vi "RTK Multiple String Capture Software.vi"() -> ()   [LabVIEW 2009]
uses:
  <vilib>/Instr/_visa.llb/VISA Configure Serial Port (Instr).vi
  <vilib>/Instr/_visa.llb/VISA Flush IO Buffer Mask.ctl
  COM Port Control.ctl
panel:
  in  "Tab Control":T1(tab)
  in  "Update setup":bool
  in  "stop":bool
  in  "Base File Path":path caption="Base File Path (Destination that all RCVR files will be saved in)"
  in  "Time between samples (seconds)":u32 max=600 step=1
  in  "Number of hours To Collect before starting new file":u16 min=1 max=24 step=1
  in  "UPDT COM 1":bool
  in  "Use RCVR 1":bool caption="Use RCVR"
  in  "Name of RCVR 1":string caption="Name of RCVR"
  in  "COM Port 1":T2 {"data bits" min=5 max=8 step=1; "flow control" items=["None", "XON/XOFF", "RTS/CTS", "XON/XOFF & RTS/CTS", "DTR/DSR", "XON/XOFF & DTR/DSR"]}
  out "Last 10 RCVR 1":string[](array[string])
  in  "Name of RCVR 2":string caption="Name of RCVR"
  in  "UPDT COM 2":bool
  out "Last 10 RCVR 2":string[](array[string])
  in  "COM Port 2":T2 {"data bits" min=5 max=8 step=1; "flow control" items=["None", "XON/XOFF", "RTS/CTS", "XON/XOFF & RTS/CTS", "DTR/DSR", "XON/XOFF & DTR/DSR"]}
  in  "Use RCVR 2":bool caption="Use RCVR"
  in  "Name of RCVR 3":string caption="Name of RCVR"
  in  "UPDT COM 3":bool
  out "Last 10 RCVR 3":string[](array[string])
  in  "COM Port 3":T2 {"data bits" min=5 max=8 step=1; "flow control" items=["None", "XON/XOFF", "RTS/CTS", "XON/XOFF & RTS/CTS", "DTR/DSR", "XON/XOFF & DTR/DSR"]}
  in  "Use RCVR 3":bool caption="Use RCVR"
  in  "Name of RCVR 4":string caption="Name of RCVR"
  in  "UPDT COM 4":bool
  out "Last 10 RCVR 4":string[](array[string])
  in  "COM Port 4":T2 {"data bits" min=5 max=8 step=1; "flow control" items=["None", "XON/XOFF", "RTS/CTS", "XON/XOFF & RTS/CTS", "DTR/DSR", "XON/XOFF & DTR/DSR"]}
  in  "Use RCVR 4":bool caption="Use RCVR"
  in  "Name of RCVR 5":string caption="Name of RCVR"
  in  "UPDT COM 5":bool
  out "Last 10 RCVR 5":string[](array[string])
  in  "COM Port 5":T2 {"data bits" min=5 max=8 step=1; "flow control" items=["None", "XON/XOFF", "RTS/CTS", "XON/XOFF & RTS/CTS", "DTR/DSR", "XON/XOFF & DTR/DSR"]}
  in  "Use RCVR 5":bool caption="Use RCVR"
  in  "Name of RCVR 6":string caption="Name of RCVR"
  in  "UPDT COM 6":bool
  out "Last 10 RCVR 6":string[](array[string])
  in  "COM Port 6":T2 {"data bits" min=5 max=8 step=1; "flow control" items=["None", "XON/XOFF", "RTS/CTS", "XON/XOFF & RTS/CTS", "DTR/DSR", "XON/XOFF & DTR/DSR"]}
  in  "Use RCVR 6":bool caption="Use RCVR"
  in  "Name of RCVR 7":string caption="Name of RCVR"
  in  "UPDT COM 7":bool
  out "Last 10 RCVR 7":string[](array[string])
  in  "COM Port 7":T2 {"data bits" min=5 max=8 step=1; "flow control" items=["None", "XON/XOFF", "RTS/CTS", "XON/XOFF & RTS/CTS", "DTR/DSR", "XON/XOFF & DTR/DSR"]}
  in  "Use RCVR 7":bool caption="Use RCVR"
  in  "Name of RCVR 8":string caption="Name of RCVR"
  in  "UPDT COM 8":bool
  out "Last 10 RCVR 8":string[](array[string])
  in  "COM Port 8":T2 {"data bits" min=5 max=8 step=1; "flow control" items=["None", "XON/XOFF", "RTS/CTS", "XON/XOFF & RTS/CTS", "DTR/DSR", "XON/XOFF & DTR/DSR"]}
  in  "Use RCVR 8":bool caption="Use RCVR"
  in  "Name of RCVR 9":string caption="Name of RCVR"
  in  "UPDT COM 9":bool
  out "Last 10 RCVR 9":string[](array[string])
  in  "COM Port 9":T2 {"data bits" min=5 max=8 step=1; "flow control" items=["None", "XON/XOFF", "RTS/CTS", "XON/XOFF & RTS/CTS", "DTR/DSR", "XON/XOFF & DTR/DSR"]}
  in  "Use RCVR 9":bool caption="Use RCVR"
  in  "Name of RCVR 10":string caption="Name of RCVR"
  in  "UPDT COM 10":bool
  out "Last 10 RCVR 10":string[](array[string])
  in  "COM Port 10":T2 {"data bits" min=5 max=8 step=1; "flow control" items=["None", "XON/XOFF", "RTS/CTS", "XON/XOFF & RTS/CTS", "DTR/DSR", "XON/XOFF & DTR/DSR"]}
  in  "Use RCVR 10":bool caption="Use RCVR"
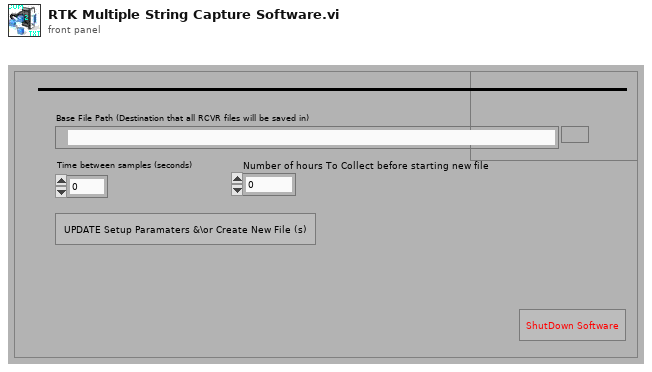
[diagram p1: front panel]
types:
  T1 = enum32{"SETUP", "RCVR 1", "RCVR 2", "RCVR 3", "RCVR 4", "RCVR 5", "RCVR 6", "RCVR 7", "RCVR 8", "RCVR 9", "RCVR 10"}
  T2 = typedef "COM Port Control.ctl" = cluster{"flow control":u16, "COM Port":refnum<visa-resource-name>, "parity":enum16{"None", "Odd", "Even", "Mark", "Space"}, "data bits":u16, "baud rate":u32}
  T3 = typedef "VISA Flush IO Buffer Mask.ctl" = u16
  T4 = enum32{"invalid app kind", "Development System", "Run Time System", "Student Edition", "Embedded LabVIEW", "Evaluation", "Custom"}
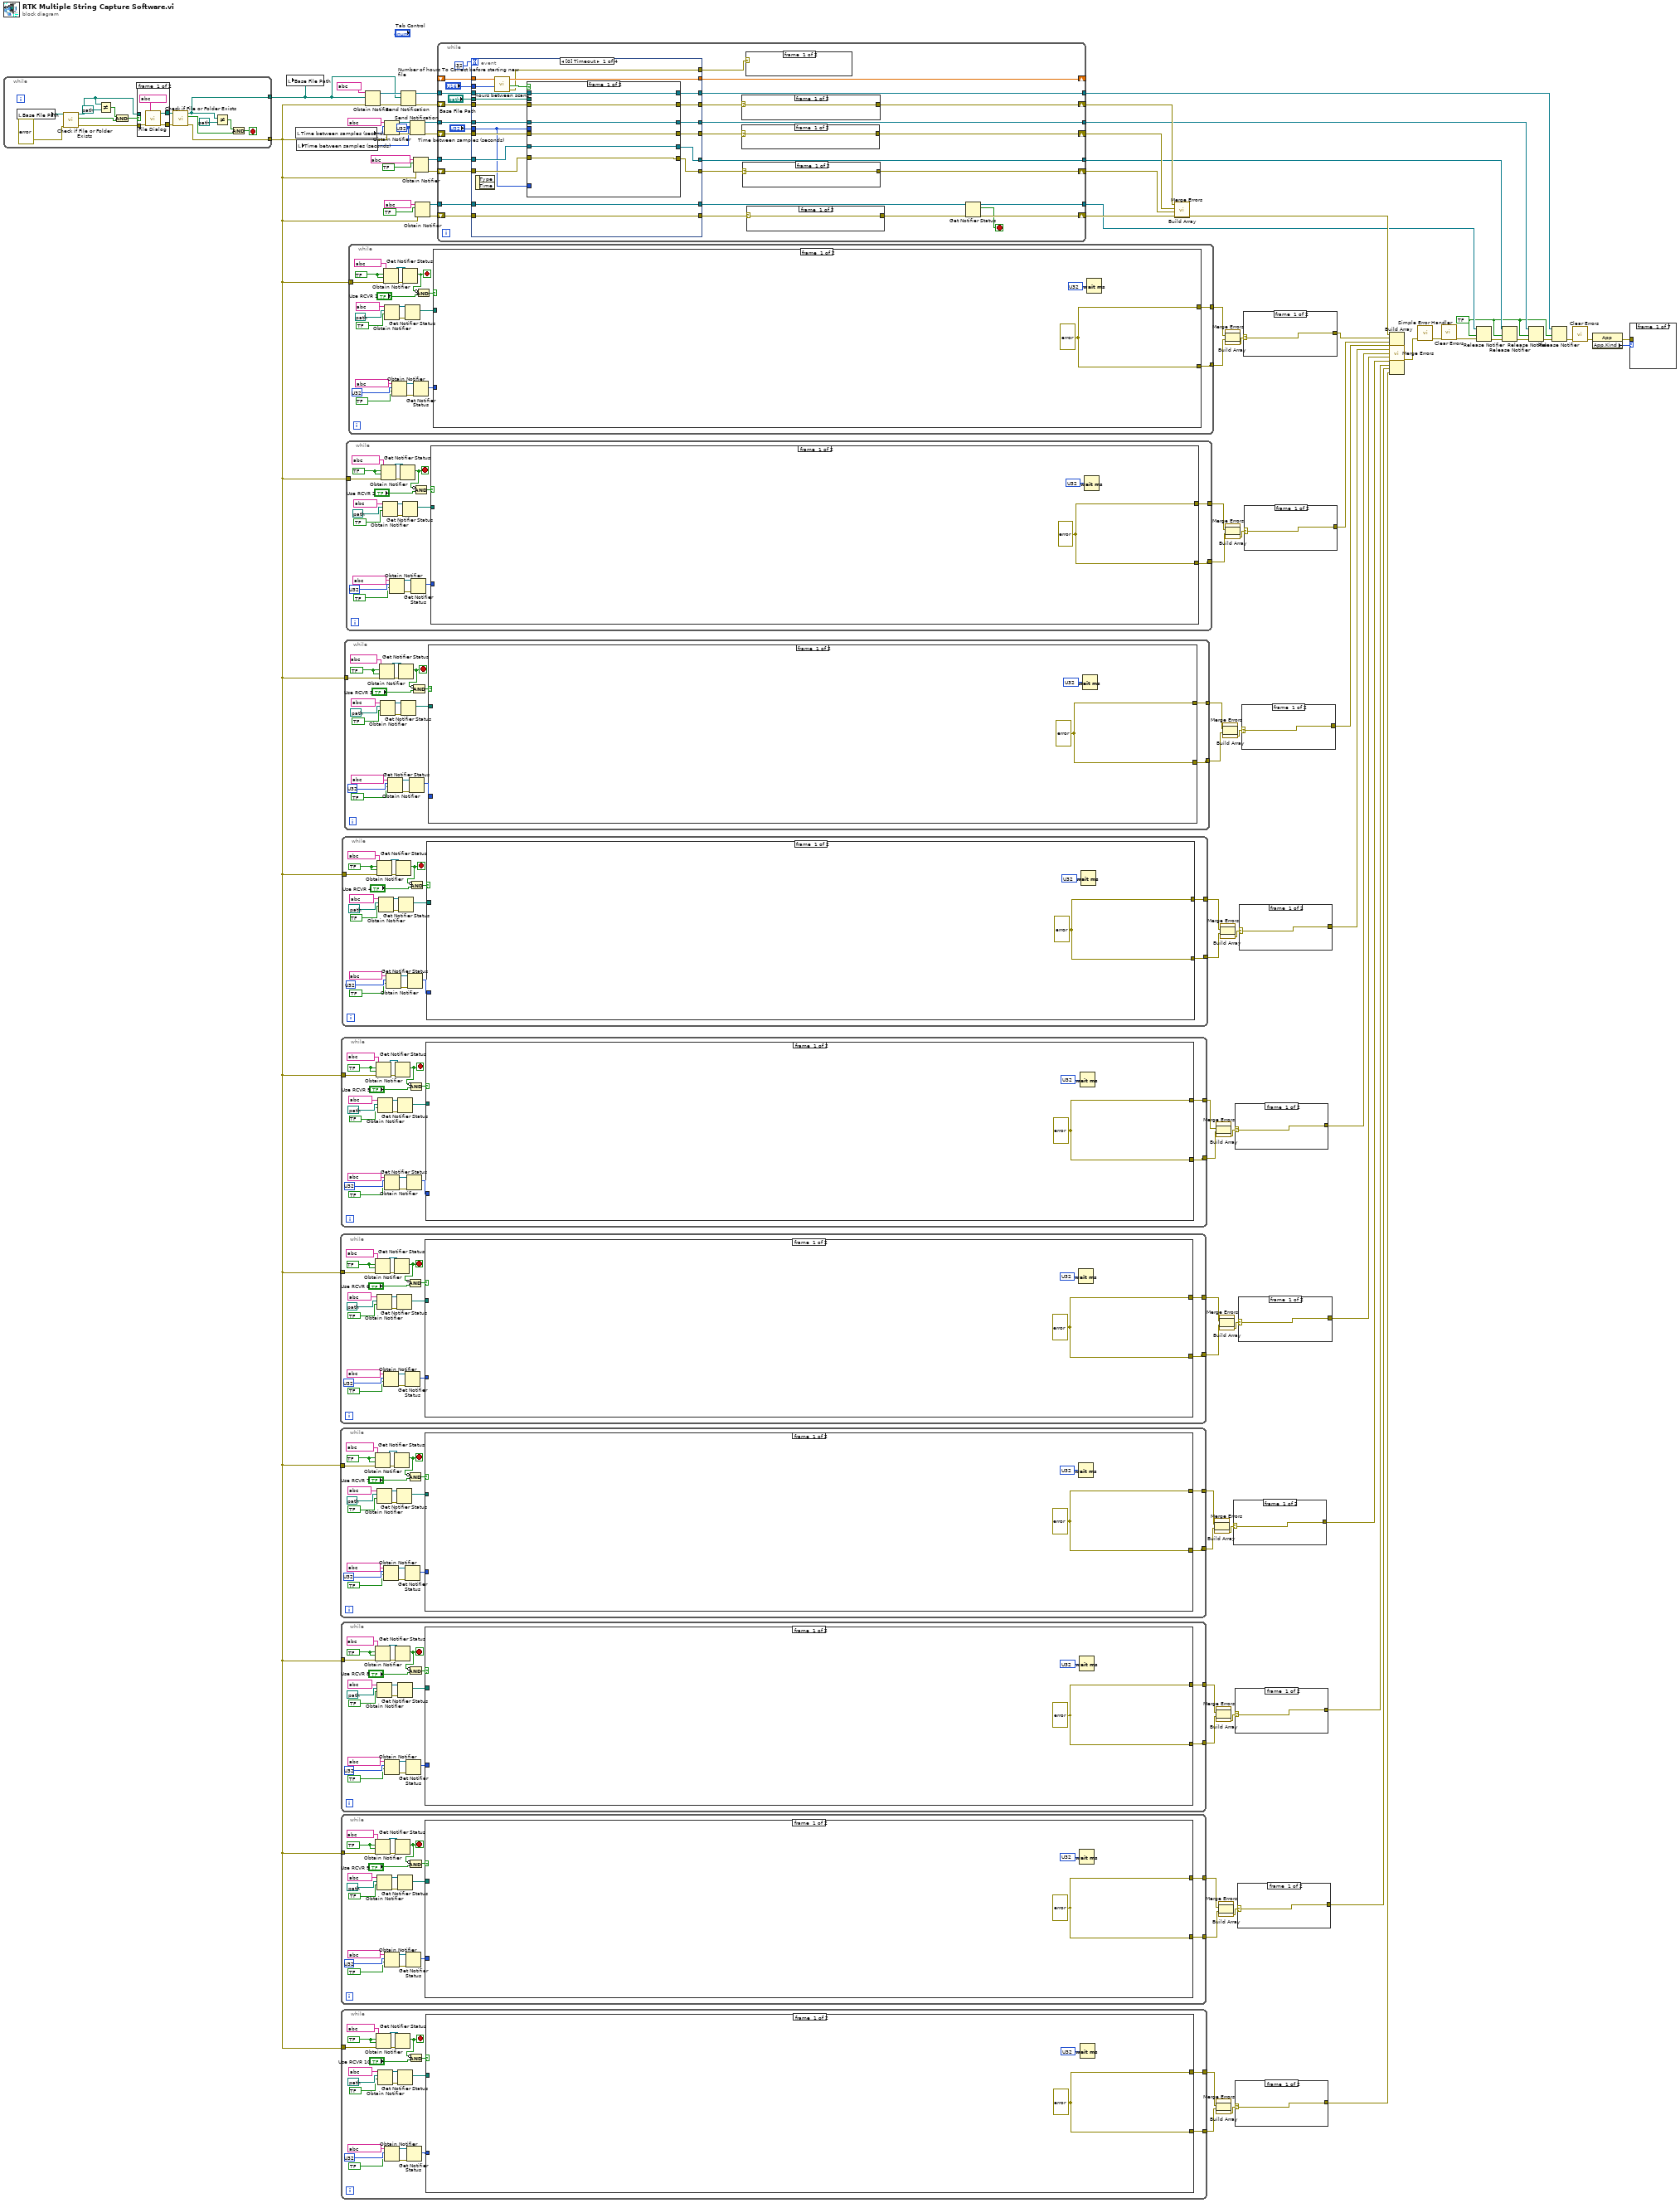
[diagram p0: block diagram]
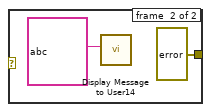
[diagram p2: hidden frame]
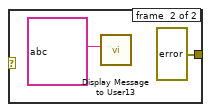
[diagram p3: hidden frame]
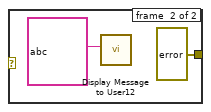
[diagram p4: hidden frame]
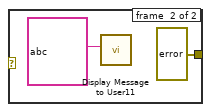
[diagram p5: hidden frame]
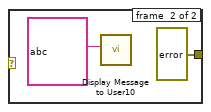
[diagram p6: hidden frame]
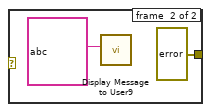
[diagram p7: hidden frame]
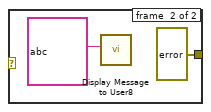
[diagram p8: hidden frame]
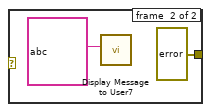
[diagram p9: hidden frame]
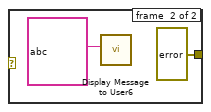
[diagram p10: hidden frame]
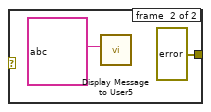
[diagram p11: hidden frame]
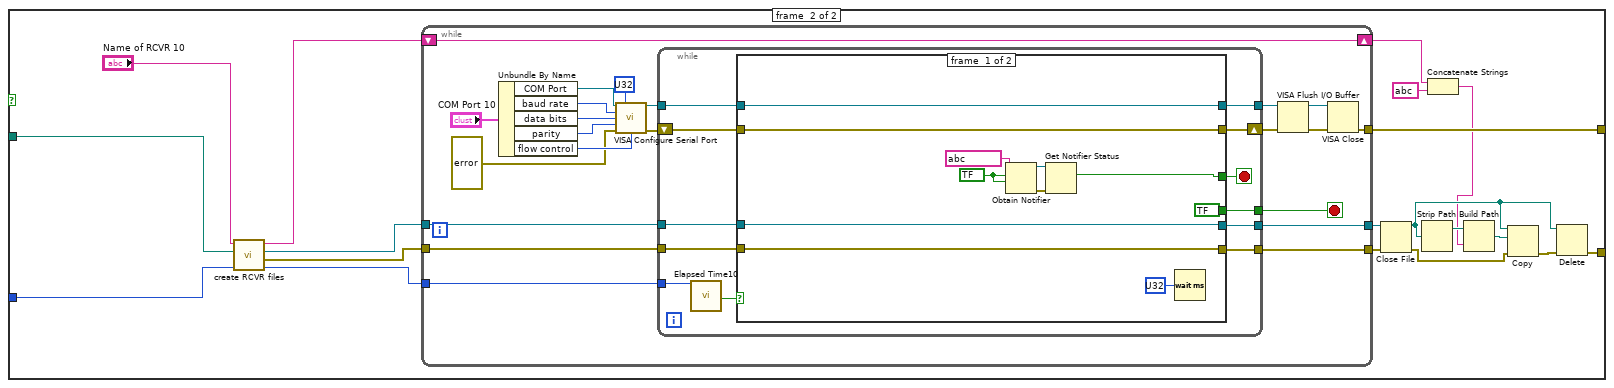
[diagram p12: hidden frame]
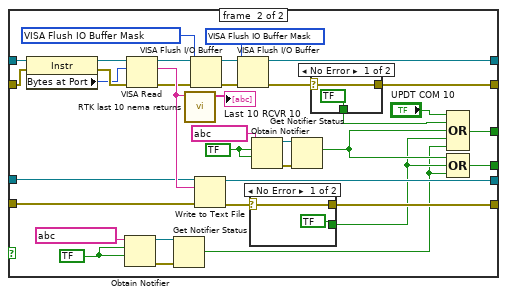
[diagram p13: hidden frame]
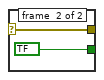
[diagram p14: hidden frame]
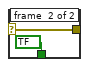
[diagram p15: hidden frame]
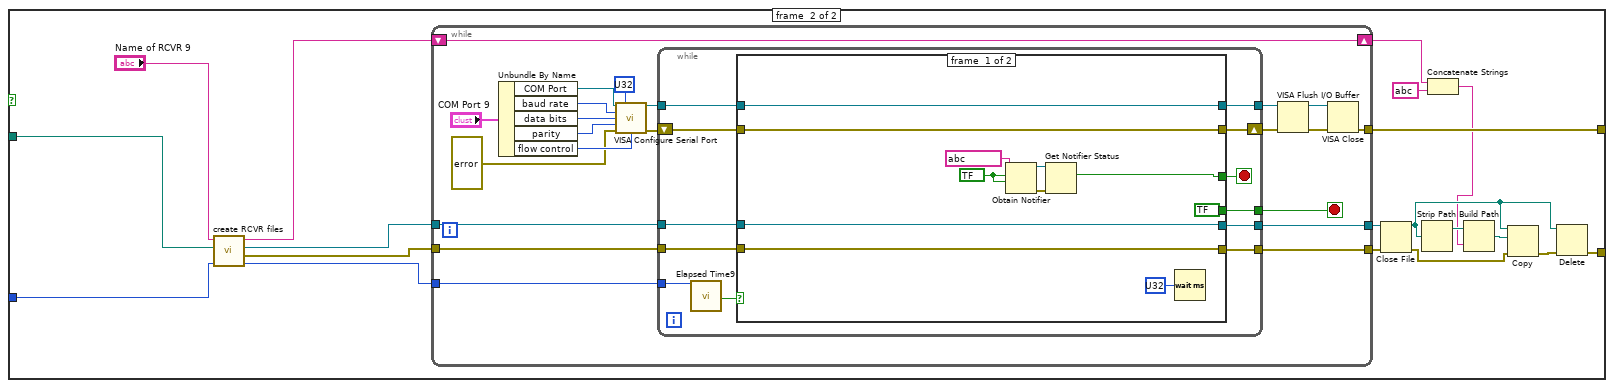
[diagram p16: hidden frame]
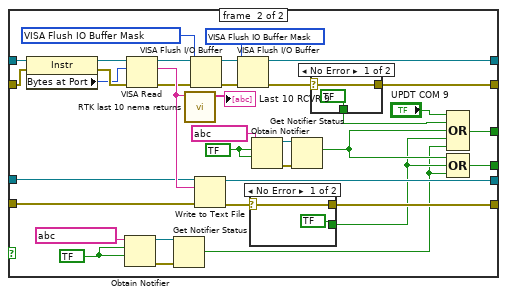
[diagram p17: hidden frame]
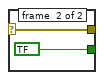
[diagram p18: hidden frame]
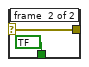
[diagram p19: hidden frame]
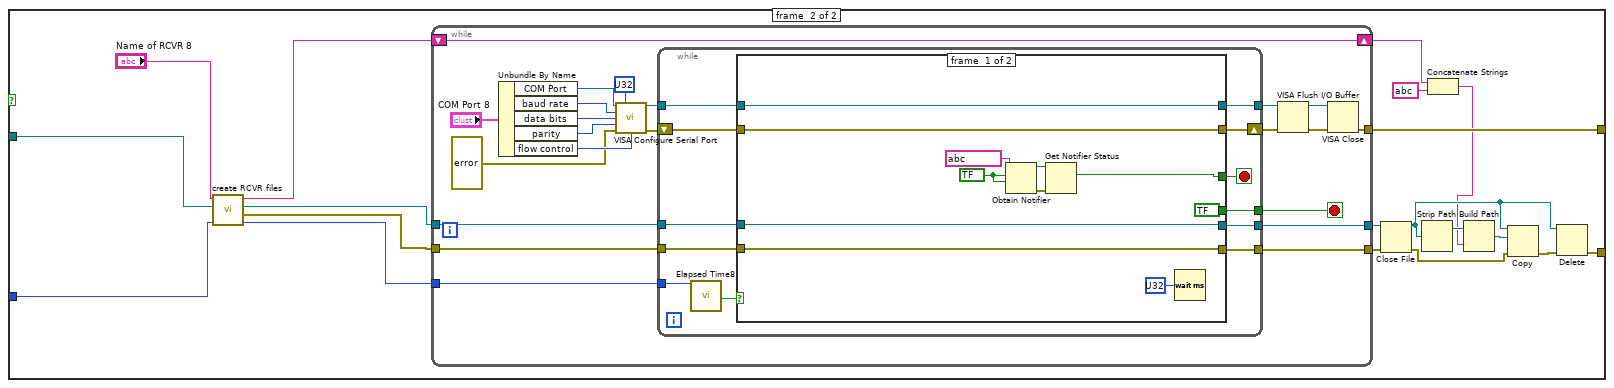
[diagram p20: hidden frame]
diagram:
  w58 = bool ?
  w73 = u32 ? ("notification")
  n1 = while {
    tunnel: [w103] -> w78
    tunnel: [w105] -> w53
    stop <- w104 stop-if-true
    n2 = local read "Base File Path"() -> (w110:path)
    n3 = call <vilib>:"Check if File or Folder Exists.vi"("error in (no error)"=errorcluster ?, "path"=w110) -> ("error out"=w107:errorcluster, "file or folder exists?"=w97:bool, "dup path"=w96:path)  [unwired: 7 in]
    n4 = Not Equal?(x=w96, y=path ?) -> (x != y?=w99:bool)
    n5 = And(x=w99, y=w97) -> (x .and. y?=w95:bool)
    n6 = case shown="True" w95 {
      tunnel: [w114 w116] -> w109
      tunnel: w96 -> [_ w116]
      tunnel: w107 -> [w113 w115]
      tunnel: [w112 w115] -> w106
      frame #0 {
        n7 = call "File Dialog"("prompt"=string ?, "error in"=w113) -> ("selected path"=w114:path, "error out"=w112:errorcluster)  [unwired: 10 in, 2 out]
      }
      frame #1 {
      }
    }
    n8 = call <vilib>:"Check if File or Folder Exists.vi"("error in (no error)"=w106, "path"=w109) -> ("error out"=w105:errorcluster, "file or folder exists?"=w100:bool, "dup path"=w103:path)  [unwired: 7 in]
    n9 = Not Equal?(x=w103, y=path ?) -> (x != y?=w101:bool)
    n10 = And(x=w101, y=w100) -> (x .and. y?=w104:bool)
  }
  n11 = local write "Base File Path"(w78) -> ()
  n12 = local read "Time between samples (seconds)"() -> (w83:u32)
  n13 = local write "Time between samples (seconds)"(w73) -> ()
  n14 = while {
    tunnel: [w120] -> w22
    tunnel: [w138] -> w23
    tunnel: w53 -> [w121]
    stop <- w119 stop-if-true
    w137 = bool ?
    n15 = Obtain Notifier(name (unnamed)=string ?, notification data type=w137, create if not found? (T)=w137, error in (no error)=w121) -> (notifier out=w134:refnum<notifier>, error out=w135:errorcluster)  [unwired: 1 out]
    n16 = Obtain Notifier(name (unnamed)=string ?, notification data type=path ?, create if not found? (T)=bool ?) -> (notifier out=w130:refnum<notifier>, error out=w131:errorcluster)  [unwired: 1 in, 1 out]
    n17 = Obtain Notifier(name (unnamed)=string ?, notification data type=u32 ?, create if not found? (T)=bool ?) -> (notifier out=w124:refnum<notifier>, error out=w125:errorcluster)  [unwired: 1 in, 1 out]
    n18 = Get Notifier Status(notifier=w134, error in (no error)=w135) -> (current notification=w119:bool)  [unwired: 4 out]
    n19 = Get Notifier Status(notifier=w130, error in (no error)=w131) -> (current notification=w129:path)  [unwired: 4 out]
    n20 = Get Notifier Status(notifier=w124, error in (no error)=w125) -> (current notification=w123:u32)  [unwired: 4 out]
    n21 = Compound Arithmetic op=AND(invert w119, "Use RCVR 6") -> (w117:bool)
    n22 = case shown="True" w117 {
      tunnel: w123 -> [_ w144]
      tunnel: [w139 w157] -> w138
      tunnel: w129 -> [_ w145]
      tunnel: [w139 w151] -> w120
      frame #0 {
        w139 = errorcluster ? ("error in (no error)")
        n23 = Wait (ms)(milliseconds to wait=u32 ?) -> ()  [unwired: 1 out]
      }
      frame #1 {
        n24 = call "create RCVR files.vi"("Sample rate in"=w144, "Save Path"=w145, "Name of RCVR 1"="Name of RCVR 6") -> ("sample rate out"=w141:u32, "error out"=w142:errorcluster, "refnum out"=w143:refnum<file>, "Name of file out"=w147:string)  [unwired: 5 in]
        n25 = while {
          tunnel: w143 -> [w181]
          tunnel: w142 -> [w180]
          tunnel: [w171] -> w159
          tunnel: [w162] -> w158
          tunnel: [w169] -> w157
          tunnel: w141 -> [w164]
          shift-right: [w160] -> w150
          shift-left: w147 -> [w160]
          stop <- w161 stop-if-true
          n26 = Unbundle By Name("COM Port 6") -> ("COM Port"=w176:refnum<visa-resource-name>, "baud rate"=w175:u32, "data bits"=w174:u16, "parity"=w173:enum16{"None", "Odd", "Even", "Mark", "Space"}, "flow control"=w172:u16)
          n27 = call-poly "VISA Configure Serial Port"("VISA resource name"=w176, "timeout (10sec)"=u32 ?, "baud rate (9600)"=w175, "data bits (8)"=w174, "parity (0:none)"=w173, "error in (no error)"=errorcluster ?, "flow control (0:none)"=w172) -> ("VISA resource name out"=w179:refnum<visa-resource-name>, "error out"=w178:errorcluster)  [unwired: 7 in]
          n28 = while {
            tunnel: [w193] -> w165
            tunnel: w181 -> [w190]
            tunnel: w180 -> [w188]
            tunnel: w179 -> [w192]
            tunnel: [w189] -> w171
            tunnel: w164 -> [w185]
            shift-right: [w187] -> w166
            shift-left: w178 -> [w191]
            tunnel: [w186] -> w162
            tunnel: [w182] -> w161
            stop <- w183 stop-if-true
            n29 = call "Elapsed Time6"("Time Target (s)"=w185) -> ("Time has Elapsed"=w184:bool)  [unwired: 11 in, 7 out]
            n30 = case shown="True" w184 {
              tunnel: [w204 w206] -> w193
              tunnel: w192 -> [w204 w240]
              tunnel: w191 -> [w203 w239]
              tunnel: w190 -> [w202 w234]
              tunnel: [w202 w233] -> w189
              tunnel: w188 -> [w201 w232]
              tunnel: [w203 w230] -> w187
              tunnel: [w197 w225] -> w183
              tunnel: [w201 w222] -> w186
              tunnel: [bool ? w214] -> w182
              frame #0 {
                w196 = bool ?
                n31 = Obtain Notifier(name (unnamed)=string ?, notification data type=w196, create if not found? (T)=w196) -> (notifier out=w200:refnum<notifier>, error out=w199:errorcluster)  [unwired: 1 in, 1 out]
                n32 = Get Notifier Status(notifier=w200, error in (no error)=w199) -> (current notification=w197:bool)  [unwired: 4 out]
                n33 = Wait (ms)(milliseconds to wait=u32 ?) -> ()  [unwired: 1 out]
              }
              frame #1 {
                w207 = T3 ? items=["Flush Receive Buffer", "Write Transmit Buffer to Device", "Flush Receive Buffer (No I/O)", "Flush Transmit Buffer"] ("Mask")
                w208 = T3 ? items=["Flush Receive Buffer", "Write Transmit Buffer to Device", "Flush Receive Buffer (No I/O)", "Flush Transmit Buffer"] ("Mask")
                w213 = bool ?
                w226 = bool ?
                n34 = property class="Instr"(reference=w240, error in=w239) -> (reference out=w238:refnum<visa-resource-name>, error out=w237:errorcluster, "Bytes at Port"=w236:u32)
                n35 = Obtain Notifier(name (unnamed)=string ?, notification data type=w213, create if not found? (T)=w213) -> (notifier out=w219:refnum<notifier>, error out=w218:errorcluster)  [unwired: 1 in, 1 out]
                n36 = VISA Read(VISA resource name=w238, byte count=w236, error in (no error)=w237) -> (VISA resource name out=w212:refnum<visa-resource-name>, read buffer=w235:string, error out=w211:errorcluster)  [unwired: 1 out]
                n37 = Get Notifier Status(notifier=w219, error in (no error)=w218) -> (current notification=w215:bool)  [unwired: 4 out]
                n38 = call "RTK last 10 nema returns.vi"("x"=w235) -> ("Array"=→"Last 10 RCVR 6":string[])  [unwired: 10 in]
                n39 = VISA Flush I/O Buffer(VISA resource name=w212, mask (16)=w208, error in (no error)=w211) -> (VISA resource name out=w209:refnum<visa-resource-name>, error out=w210:errorcluster)
                n40 = Write to Text File(file (use dialog)=w234, text=w235, error in=w232) -> (refnum out=w233:refnum<file>, error out=w223:errorcluster)  [unwired: 1 in, 1 out]
                n41 = VISA Flush I/O Buffer(VISA resource name=w209, mask (16)=w207, error in (no error)=w210) -> (VISA resource name out=w206:refnum<visa-resource-name>, error out=w205:errorcluster)
                n42 = case shown="No Error" w223 {
                  selector: w223 -> [w241 w243]
                  tunnel: [bool ? bool ?] -> w216
                  tunnel: [w241 w243] -> w222
                  frame #0 {
                  }
                  frame #1 {
                  }
                }
                n43 = Obtain Notifier(name (unnamed)=string ?, notification data type=w226, create if not found? (T)=w226) -> (notifier out=w229:refnum<notifier>, error out=w228:errorcluster)  [unwired: 1 in, 1 out]
                n44 = Get Notifier Status(notifier=w229, error in (no error)=w228) -> (current notification=w217:bool)  [unwired: 4 out]
                n45 = case shown="No Error" w205 {
                  selector: w205 -> [w245 w247]
                  tunnel: [bool ? bool ?] -> w224
                  tunnel: [w245 w247] -> w230
                  frame #0 {
                  }
                  frame #1 {
                  }
                }
                n46 = Compound Arithmetic op=OR("UPDT COM 6", w224, w217, w216, w215) -> (w225:bool)
                n47 = Compound Arithmetic op=OR(w217, w216, w215) -> (w214:bool)
              }
            }
          }
          n48 = VISA Flush I/O Buffer(VISA resource name=w165, error in (no error)=w166) -> (VISA resource name out=w168:refnum<visa-resource-name>, error out=w167:errorcluster)  [unwired: 1 in]
          n49 = VISA Close(VISA resource name=w168, error in (no error)=w167) -> (error out=w169:errorcluster)
        }
        n50 = Close File(refnum=w159, error in=w158) -> (path=w152:path, error out=w153:errorcluster)
        n51 = Strip Path(path=w152) -> (stripped path=w155:path)  [unwired: 1 out]
        n52 = Concatenate Strings(w150, string ? ("string")) -> (w148:string)
        n53 = Build Path(base path=w155, name or relative path=w148) -> (appended path=w156:path)
        n54 = Copy(8:w153, 10:w156, 11:w152) -> (0:w154:errorcluster)  [unwired: 2 in, 2 out]
        n55 = Delete(path (use dialog)=w152, error in=w154) -> (error out=w151:errorcluster)  [unwired: 3 in, 2 out]
      }
    }
  }
  n56 = while {
    tunnel: [w252] -> w19
    tunnel: [w270] -> w20
    tunnel: w53 -> [w253]
    stop <- w251 stop-if-true
    w269 = bool ?
    n57 = Obtain Notifier(name (unnamed)=string ?, notification data type=w269, create if not found? (T)=w269, error in (no error)=w253) -> (notifier out=w266:refnum<notifier>, error out=w267:errorcluster)  [unwired: 1 out]
    n58 = Obtain Notifier(name (unnamed)=string ?, notification data type=path ?, create if not found? (T)=bool ?) -> (notifier out=w262:refnum<notifier>, error out=w263:errorcluster)  [unwired: 1 in, 1 out]
    n59 = Obtain Notifier(name (unnamed)=string ?, notification data type=u32 ?, create if not found? (T)=bool ?) -> (notifier out=w256:refnum<notifier>, error out=w257:errorcluster)  [unwired: 1 in, 1 out]
    n60 = Get Notifier Status(notifier=w266, error in (no error)=w267) -> (current notification=w251:bool)  [unwired: 4 out]
    n61 = Get Notifier Status(notifier=w262, error in (no error)=w263) -> (current notification=w261:path)  [unwired: 4 out]
    n62 = Get Notifier Status(notifier=w256, error in (no error)=w257) -> (current notification=w255:u32)  [unwired: 4 out]
    n63 = Compound Arithmetic op=AND(invert w251, "Use RCVR 7") -> (w249:bool)
    n64 = case shown="True" w249 {
      tunnel: w255 -> [_ w273]
      tunnel: [w271 w289] -> w270
      tunnel: w261 -> [_ w274]
      tunnel: [w271 w283] -> w252
      frame #0 {
        w271 = errorcluster ? ("error in (no error)")
        n65 = Wait (ms)(milliseconds to wait=u32 ?) -> ()  [unwired: 1 out]
      }
      frame #1 {
        n66 = call "create RCVR files.vi"("Sample rate in"=w273, "Save Path"=w274, "Name of RCVR 1"="Name of RCVR 7") -> ("sample rate out"=w276:u32, "error out"=w277:errorcluster, "refnum out"=w278:refnum<file>, "Name of file out"=w279:string)  [unwired: 5 in]
        n67 = while {
          tunnel: w278 -> [w313]
          tunnel: w277 -> [w312]
          tunnel: [w303] -> w291
          tunnel: [w294] -> w290
          tunnel: [w301] -> w289
          tunnel: w276 -> [w296]
          shift-right: [w292] -> w282
          shift-left: w279 -> [w292]
          stop <- w293 stop-if-true
          n68 = Unbundle By Name("COM Port 7") -> ("COM Port"=w308:refnum<visa-resource-name>, "baud rate"=w307:u32, "data bits"=w306:u16, "parity"=w305:enum16{"None", "Odd", "Even", "Mark", "Space"}, "flow control"=w304:u16)
          n69 = call-poly "VISA Configure Serial Port"("VISA resource name"=w308, "timeout (10sec)"=u32 ?, "baud rate (9600)"=w307, "data bits (8)"=w306, "parity (0:none)"=w305, "error in (no error)"=errorcluster ?, "flow control (0:none)"=w304) -> ("VISA resource name out"=w311:refnum<visa-resource-name>, "error out"=w310:errorcluster)  [unwired: 7 in]
          n70 = while {
            tunnel: [w325] -> w297
            tunnel: w313 -> [w322]
            tunnel: w312 -> [w320]
            tunnel: w311 -> [w324]
            tunnel: [w321] -> w303
            tunnel: w296 -> [w317]
            shift-right: [w319] -> w298
            shift-left: w310 -> [w323]
            tunnel: [w318] -> w294
            tunnel: [w314] -> w293
            stop <- w315 stop-if-true
            n71 = call "Elapsed Time7"("Time Target (s)"=w317) -> ("Time has Elapsed"=w316:bool)  [unwired: 11 in, 7 out]
            n72 = case shown="True" w316 {
              tunnel: [w336 w338] -> w325
              tunnel: w324 -> [w336 w372]
              tunnel: w323 -> [w335 w371]
              tunnel: w322 -> [w334 w366]
              tunnel: [w334 w365] -> w321
              tunnel: w320 -> [w333 w364]
              tunnel: [w335 w362] -> w319
              tunnel: [w329 w357] -> w315
              tunnel: [w333 w354] -> w318
              tunnel: [bool ? w346] -> w314
              frame #0 {
                w328 = bool ?
                n73 = Obtain Notifier(name (unnamed)=string ?, notification data type=w328, create if not found? (T)=w328) -> (notifier out=w332:refnum<notifier>, error out=w331:errorcluster)  [unwired: 1 in, 1 out]
                n74 = Get Notifier Status(notifier=w332, error in (no error)=w331) -> (current notification=w329:bool)  [unwired: 4 out]
                n75 = Wait (ms)(milliseconds to wait=u32 ?) -> ()  [unwired: 1 out]
              }
              frame #1 {
                w339 = T3 ? items=["Flush Receive Buffer", "Write Transmit Buffer to Device", "Flush Receive Buffer (No I/O)", "Flush Transmit Buffer"] ("Mask")
                w340 = T3 ? items=["Flush Receive Buffer", "Write Transmit Buffer to Device", "Flush Receive Buffer (No I/O)", "Flush Transmit Buffer"] ("Mask")
                w345 = bool ?
                w358 = bool ?
                n76 = property class="Instr"(reference=w372, error in=w371) -> (reference out=w370:refnum<visa-resource-name>, error out=w369:errorcluster, "Bytes at Port"=w368:u32)
                n77 = Obtain Notifier(name (unnamed)=string ?, notification data type=w345, create if not found? (T)=w345) -> (notifier out=w351:refnum<notifier>, error out=w350:errorcluster)  [unwired: 1 in, 1 out]
                n78 = VISA Read(VISA resource name=w370, byte count=w368, error in (no error)=w369) -> (VISA resource name out=w344:refnum<visa-resource-name>, read buffer=w367:string, error out=w343:errorcluster)  [unwired: 1 out]
                n79 = Get Notifier Status(notifier=w351, error in (no error)=w350) -> (current notification=w347:bool)  [unwired: 4 out]
                n80 = call "RTK last 10 nema returns.vi"("x"=w367) -> ("Array"=→"Last 10 RCVR 7":string[])  [unwired: 10 in]
                n81 = VISA Flush I/O Buffer(VISA resource name=w344, mask (16)=w340, error in (no error)=w343) -> (VISA resource name out=w341:refnum<visa-resource-name>, error out=w342:errorcluster)
                n82 = Write to Text File(file (use dialog)=w366, text=w367, error in=w364) -> (refnum out=w365:refnum<file>, error out=w355:errorcluster)  [unwired: 1 in, 1 out]
                n83 = VISA Flush I/O Buffer(VISA resource name=w341, mask (16)=w339, error in (no error)=w342) -> (VISA resource name out=w338:refnum<visa-resource-name>, error out=w337:errorcluster)
                n84 = case shown="No Error" w355 {
                  selector: w355 -> [w373 w375]
                  tunnel: [bool ? bool ?] -> w348
                  tunnel: [w373 w375] -> w354
                  frame #0 {
                  }
                  frame #1 {
                  }
                }
                n85 = Obtain Notifier(name (unnamed)=string ?, notification data type=w358, create if not found? (T)=w358) -> (notifier out=w361:refnum<notifier>, error out=w360:errorcluster)  [unwired: 1 in, 1 out]
                n86 = Get Notifier Status(notifier=w361, error in (no error)=w360) -> (current notification=w349:bool)  [unwired: 4 out]
                n87 = case shown="No Error" w337 {
                  selector: w337 -> [w377 w379]
                  tunnel: [bool ? bool ?] -> w356
                  tunnel: [w377 w379] -> w362
                  frame #0 {
                  }
                  frame #1 {
                  }
                }
                n88 = Compound Arithmetic op=OR("UPDT COM 7", w356, w349, w348, w347) -> (w357:bool)
                n89 = Compound Arithmetic op=OR(w349, w348, w347) -> (w346:bool)
              }
            }
          }
          n90 = VISA Flush I/O Buffer(VISA resource name=w297, error in (no error)=w298) -> (VISA resource name out=w300:refnum<visa-resource-name>, error out=w299:errorcluster)  [unwired: 1 in]
          n91 = VISA Close(VISA resource name=w300, error in (no error)=w299) -> (error out=w301:errorcluster)
        }
        n92 = Close File(refnum=w291, error in=w290) -> (path=w284:path, error out=w285:errorcluster)
        n93 = Strip Path(path=w284) -> (stripped path=w287:path)  [unwired: 1 out]
        n94 = Concatenate Strings(w282, string ? ("string")) -> (w280:string)
        n95 = Build Path(base path=w287, name or relative path=w280) -> (appended path=w288:path)
        n96 = Copy(8:w285, 10:w288, 11:w284) -> (0:w286:errorcluster)  [unwired: 2 in, 2 out]
        n97 = Delete(path (use dialog)=w284, error in=w286) -> (error out=w283:errorcluster)  [unwired: 3 in, 2 out]
      }
    }
  }
  n98 = while {
    tunnel: [w384] -> w16
    tunnel: [w402] -> w17
    tunnel: w53 -> [w385]
    stop <- w383 stop-if-true
    w401 = bool ?
    n99 = Obtain Notifier(name (unnamed)=string ?, notification data type=w401, create if not found? (T)=w401, error in (no error)=w385) -> (notifier out=w398:refnum<notifier>, error out=w399:errorcluster)  [unwired: 1 out]
    n100 = Obtain Notifier(name (unnamed)=string ?, notification data type=path ?, create if not found? (T)=bool ?) -> (notifier out=w394:refnum<notifier>, error out=w395:errorcluster)  [unwired: 1 in, 1 out]
    n101 = Obtain Notifier(name (unnamed)=string ?, notification data type=u32 ?, create if not found? (T)=bool ?) -> (notifier out=w388:refnum<notifier>, error out=w389:errorcluster)  [unwired: 1 in, 1 out]
    n102 = Get Notifier Status(notifier=w398, error in (no error)=w399) -> (current notification=w383:bool)  [unwired: 4 out]
    n103 = Get Notifier Status(notifier=w394, error in (no error)=w395) -> (current notification=w393:path)  [unwired: 4 out]
    n104 = Get Notifier Status(notifier=w388, error in (no error)=w389) -> (current notification=w387:u32)  [unwired: 4 out]
    n105 = Compound Arithmetic op=AND(invert w383, "Use RCVR 8") -> (w381:bool)
    n106 = case shown="True" w381 {
      tunnel: w387 -> [_ w405]
      tunnel: [w403 w421] -> w402
      tunnel: w393 -> [_ w406]
      tunnel: [w403 w415] -> w384
      frame #0 {
        w403 = errorcluster ? ("error in (no error)")
        n107 = Wait (ms)(milliseconds to wait=u32 ?) -> ()  [unwired: 1 out]
      }
      frame #1 {
        n108 = call "create RCVR files.vi"("Sample rate in"=w405, "Save Path"=w406, "Name of RCVR 1"="Name of RCVR 8") -> ("sample rate out"=w408:u32, "error out"=w409:errorcluster, "refnum out"=w410:refnum<file>, "Name of file out"=w411:string)  [unwired: 5 in]
        n109 = while {
          tunnel: w410 -> [w445]
          tunnel: w409 -> [w444]
          tunnel: [w435] -> w423
          tunnel: [w426] -> w422
          tunnel: [w433] -> w421
          tunnel: w408 -> [w428]
          shift-right: [w424] -> w414
          shift-left: w411 -> [w424]
          stop <- w425 stop-if-true
          n110 = Unbundle By Name("COM Port 8") -> ("COM Port"=w440:refnum<visa-resource-name>, "baud rate"=w439:u32, "data bits"=w438:u16, "parity"=w437:enum16{"None", "Odd", "Even", "Mark", "Space"}, "flow control"=w436:u16)
          n111 = call-poly "VISA Configure Serial Port"("VISA resource name"=w440, "timeout (10sec)"=u32 ?, "baud rate (9600)"=w439, "data bits (8)"=w438, "parity (0:none)"=w437, "error in (no error)"=errorcluster ?, "flow control (0:none)"=w436) -> ("VISA resource name out"=w443:refnum<visa-resource-name>, "error out"=w442:errorcluster)  [unwired: 7 in]
          n112 = while {
            tunnel: [w457] -> w429
            tunnel: w445 -> [w454]
            tunnel: w444 -> [w452]
            tunnel: w443 -> [w456]
            tunnel: [w453] -> w435
            tunnel: w428 -> [w449]
            shift-right: [w451] -> w430
            shift-left: w442 -> [w455]
            tunnel: [w450] -> w426
            tunnel: [w446] -> w425
            stop <- w447 stop-if-true
            n113 = call "Elapsed Time8"("Time Target (s)"=w449) -> ("Time has Elapsed"=w448:bool)  [unwired: 11 in, 7 out]
            n114 = case shown="True" w448 {
              tunnel: [w468 w470] -> w457
              tunnel: w456 -> [w468 w504]
              tunnel: w455 -> [w467 w503]
              tunnel: w454 -> [w466 w498]
              tunnel: [w466 w497] -> w453
              tunnel: w452 -> [w465 w496]
              tunnel: [w467 w494] -> w451
              tunnel: [w461 w489] -> w447
              tunnel: [w465 w486] -> w450
              tunnel: [bool ? w478] -> w446
              frame #0 {
                w460 = bool ?
                n115 = Obtain Notifier(name (unnamed)=string ?, notification data type=w460, create if not found? (T)=w460) -> (notifier out=w464:refnum<notifier>, error out=w463:errorcluster)  [unwired: 1 in, 1 out]
                n116 = Get Notifier Status(notifier=w464, error in (no error)=w463) -> (current notification=w461:bool)  [unwired: 4 out]
                n117 = Wait (ms)(milliseconds to wait=u32 ?) -> ()  [unwired: 1 out]
              }
              frame #1 {
                w471 = T3 ? items=["Flush Receive Buffer", "Write Transmit Buffer to Device", "Flush Receive Buffer (No I/O)", "Flush Transmit Buffer"] ("Mask")
                w472 = T3 ? items=["Flush Receive Buffer", "Write Transmit Buffer to Device", "Flush Receive Buffer (No I/O)", "Flush Transmit Buffer"] ("Mask")
                w477 = bool ?
                w490 = bool ?
                n118 = property class="Instr"(reference=w504, error in=w503) -> (reference out=w502:refnum<visa-resource-name>, error out=w501:errorcluster, "Bytes at Port"=w500:u32)
                n119 = Obtain Notifier(name (unnamed)=string ?, notification data type=w477, create if not found? (T)=w477) -> (notifier out=w483:refnum<notifier>, error out=w482:errorcluster)  [unwired: 1 in, 1 out]
                n120 = VISA Read(VISA resource name=w502, byte count=w500, error in (no error)=w501) -> (VISA resource name out=w476:refnum<visa-resource-name>, read buffer=w499:string, error out=w475:errorcluster)  [unwired: 1 out]
                n121 = Get Notifier Status(notifier=w483, error in (no error)=w482) -> (current notification=w479:bool)  [unwired: 4 out]
                n122 = call "RTK last 10 nema returns.vi"("x"=w499) -> ("Array"=→"Last 10 RCVR 8":string[])  [unwired: 10 in]
                n123 = VISA Flush I/O Buffer(VISA resource name=w476, mask (16)=w472, error in (no error)=w475) -> (VISA resource name out=w473:refnum<visa-resource-name>, error out=w474:errorcluster)
                n124 = Write to Text File(file (use dialog)=w498, text=w499, error in=w496) -> (refnum out=w497:refnum<file>, error out=w487:errorcluster)  [unwired: 1 in, 1 out]
                n125 = VISA Flush I/O Buffer(VISA resource name=w473, mask (16)=w471, error in (no error)=w474) -> (VISA resource name out=w470:refnum<visa-resource-name>, error out=w469:errorcluster)
                n126 = case shown="No Error" w487 {
                  selector: w487 -> [w505 w507]
                  tunnel: [bool ? bool ?] -> w480
                  tunnel: [w505 w507] -> w486
                  frame #0 {
                  }
                  frame #1 {
                  }
                }
                n127 = Obtain Notifier(name (unnamed)=string ?, notification data type=w490, create if not found? (T)=w490) -> (notifier out=w493:refnum<notifier>, error out=w492:errorcluster)  [unwired: 1 in, 1 out]
                n128 = Get Notifier Status(notifier=w493, error in (no error)=w492) -> (current notification=w481:bool)  [unwired: 4 out]
                n129 = case shown="No Error" w469 {
                  selector: w469 -> [w509 w511]
                  tunnel: [bool ? bool ?] -> w488
                  tunnel: [w509 w511] -> w494
                  frame #0 {
                  }
                  frame #1 {
                  }
                }
                n130 = Compound Arithmetic op=OR("UPDT COM 8", w488, w481, w480, w479) -> (w489:bool)
                n131 = Compound Arithmetic op=OR(w481, w480, w479) -> (w478:bool)
              }
            }
          }
          n132 = VISA Flush I/O Buffer(VISA resource name=w429, error in (no error)=w430) -> (VISA resource name out=w432:refnum<visa-resource-name>, error out=w431:errorcluster)  [unwired: 1 in]
          n133 = VISA Close(VISA resource name=w432, error in (no error)=w431) -> (error out=w433:errorcluster)
        }
        n134 = Close File(refnum=w423, error in=w422) -> (path=w416:path, error out=w417:errorcluster)
        n135 = Strip Path(path=w416) -> (stripped path=w419:path)  [unwired: 1 out]
        n136 = Concatenate Strings(w414, string ? ("string")) -> (w412:string)
        n137 = Build Path(base path=w419, name or relative path=w412) -> (appended path=w420:path)
        n138 = Copy(8:w417, 10:w420, 11:w416) -> (0:w418:errorcluster)  [unwired: 2 in, 2 out]
        n139 = Delete(path (use dialog)=w416, error in=w418) -> (error out=w415:errorcluster)  [unwired: 3 in, 2 out]
      }
    }
  }
  n140 = while {
    tunnel: [w516] -> w47
    tunnel: [w534] -> w48
    tunnel: w53 -> [w517]
    stop <- w515 stop-if-true
    w533 = bool ?
    n141 = Obtain Notifier(name (unnamed)=string ?, notification data type=w533, create if not found? (T)=w533, error in (no error)=w517) -> (notifier out=w530:refnum<notifier>, error out=w531:errorcluster)  [unwired: 1 out]
    n142 = Obtain Notifier(name (unnamed)=string ?, notification data type=path ?, create if not found? (T)=bool ?) -> (notifier out=w526:refnum<notifier>, error out=w527:errorcluster)  [unwired: 1 in, 1 out]
    n143 = Obtain Notifier(name (unnamed)=string ?, notification data type=u32 ?, create if not found? (T)=bool ?) -> (notifier out=w520:refnum<notifier>, error out=w521:errorcluster)  [unwired: 1 in, 1 out]
    n144 = Get Notifier Status(notifier=w530, error in (no error)=w531) -> (current notification=w515:bool)  [unwired: 4 out]
    n145 = Get Notifier Status(notifier=w526, error in (no error)=w527) -> (current notification=w525:path)  [unwired: 4 out]
    n146 = Get Notifier Status(notifier=w520, error in (no error)=w521) -> (current notification=w519:u32)  [unwired: 4 out]
    n147 = Compound Arithmetic op=AND(invert w515, "Use RCVR 9") -> (w513:bool)
    n148 = case shown="True" w513 {
      tunnel: w519 -> [_ w537]
      tunnel: [w535 w553] -> w534
      tunnel: w525 -> [_ w538]
      tunnel: [w535 w547] -> w516
      frame #0 {
        w535 = errorcluster ? ("error in (no error)")
        n149 = Wait (ms)(milliseconds to wait=u32 ?) -> ()  [unwired: 1 out]
      }
      frame #1 {
        n150 = call "create RCVR files.vi"("Sample rate in"=w537, "Save Path"=w538, "Name of RCVR 1"="Name of RCVR 9") -> ("sample rate out"=w540:u32, "error out"=w541:errorcluster, "refnum out"=w542:refnum<file>, "Name of file out"=w543:string)  [unwired: 5 in]
        n151 = while {
          tunnel: w542 -> [w577]
          tunnel: w541 -> [w576]
          tunnel: [w567] -> w555
          tunnel: [w558] -> w554
          tunnel: [w565] -> w553
          tunnel: w540 -> [w560]
          shift-right: [w556] -> w546
          shift-left: w543 -> [w556]
          stop <- w557 stop-if-true
          n152 = Unbundle By Name("COM Port 9") -> ("COM Port"=w572:refnum<visa-resource-name>, "baud rate"=w571:u32, "data bits"=w570:u16, "parity"=w569:enum16{"None", "Odd", "Even", "Mark", "Space"}, "flow control"=w568:u16)
          n153 = call-poly "VISA Configure Serial Port"("VISA resource name"=w572, "timeout (10sec)"=u32 ?, "baud rate (9600)"=w571, "data bits (8)"=w570, "parity (0:none)"=w569, "error in (no error)"=errorcluster ?, "flow control (0:none)"=w568) -> ("VISA resource name out"=w575:refnum<visa-resource-name>, "error out"=w574:errorcluster)  [unwired: 7 in]
          n154 = while {
            tunnel: [w589] -> w561
            tunnel: w577 -> [w586]
            tunnel: w576 -> [w584]
            tunnel: w575 -> [w588]
            tunnel: [w585] -> w567
            tunnel: w560 -> [w581]
            shift-right: [w583] -> w562
            shift-left: w574 -> [w587]
            tunnel: [w582] -> w558
            tunnel: [w578] -> w557
            stop <- w579 stop-if-true
            n155 = call "Elapsed Time9"("Time Target (s)"=w581) -> ("Time has Elapsed"=w580:bool)  [unwired: 11 in, 7 out]
            n156 = case shown="True" w580 {
              tunnel: [w600 w602] -> w589
              tunnel: w588 -> [w600 w636]
              tunnel: w587 -> [w599 w635]
              tunnel: w586 -> [w598 w630]
              tunnel: [w598 w629] -> w585
              tunnel: w584 -> [w597 w628]
              tunnel: [w599 w626] -> w583
              tunnel: [w593 w621] -> w579
              tunnel: [w597 w618] -> w582
              tunnel: [bool ? w610] -> w578
              frame #0 {
                w592 = bool ?
                n157 = Obtain Notifier(name (unnamed)=string ?, notification data type=w592, create if not found? (T)=w592) -> (notifier out=w596:refnum<notifier>, error out=w595:errorcluster)  [unwired: 1 in, 1 out]
                n158 = Get Notifier Status(notifier=w596, error in (no error)=w595) -> (current notification=w593:bool)  [unwired: 4 out]
                n159 = Wait (ms)(milliseconds to wait=u32 ?) -> ()  [unwired: 1 out]
              }
              frame #1 {
                w603 = T3 ? items=["Flush Receive Buffer", "Write Transmit Buffer to Device", "Flush Receive Buffer (No I/O)", "Flush Transmit Buffer"] ("Mask")
                w604 = T3 ? items=["Flush Receive Buffer", "Write Transmit Buffer to Device", "Flush Receive Buffer (No I/O)", "Flush Transmit Buffer"] ("Mask")
                w609 = bool ?
                w622 = bool ?
                n160 = property class="Instr"(reference=w636, error in=w635) -> (reference out=w634:refnum<visa-resource-name>, error out=w633:errorcluster, "Bytes at Port"=w632:u32)
                n161 = Obtain Notifier(name (unnamed)=string ?, notification data type=w609, create if not found? (T)=w609) -> (notifier out=w615:refnum<notifier>, error out=w614:errorcluster)  [unwired: 1 in, 1 out]
                n162 = VISA Read(VISA resource name=w634, byte count=w632, error in (no error)=w633) -> (VISA resource name out=w608:refnum<visa-resource-name>, read buffer=w631:string, error out=w607:errorcluster)  [unwired: 1 out]
                n163 = Get Notifier Status(notifier=w615, error in (no error)=w614) -> (current notification=w611:bool)  [unwired: 4 out]
                n164 = call "RTK last 10 nema returns.vi"("x"=w631) -> ("Array"=→"Last 10 RCVR 9":string[])  [unwired: 10 in]
                n165 = VISA Flush I/O Buffer(VISA resource name=w608, mask (16)=w604, error in (no error)=w607) -> (VISA resource name out=w605:refnum<visa-resource-name>, error out=w606:errorcluster)
                n166 = Write to Text File(file (use dialog)=w630, text=w631, error in=w628) -> (refnum out=w629:refnum<file>, error out=w619:errorcluster)  [unwired: 1 in, 1 out]
                n167 = VISA Flush I/O Buffer(VISA resource name=w605, mask (16)=w603, error in (no error)=w606) -> (VISA resource name out=w602:refnum<visa-resource-name>, error out=w601:errorcluster)
                n168 = case shown="No Error" w619 {
                  selector: w619 -> [w637 w639]
                  tunnel: [bool ? bool ?] -> w612
                  tunnel: [w637 w639] -> w618
                  frame #0 {
                  }
                  frame #1 {
                  }
                }
                n169 = Obtain Notifier(name (unnamed)=string ?, notification data type=w622, create if not found? (T)=w622) -> (notifier out=w625:refnum<notifier>, error out=w624:errorcluster)  [unwired: 1 in, 1 out]
                n170 = Get Notifier Status(notifier=w625, error in (no error)=w624) -> (current notification=w613:bool)  [unwired: 4 out]
                n171 = case shown="No Error" w601 {
                  selector: w601 -> [w641 w643]
                  tunnel: [bool ? bool ?] -> w620
                  tunnel: [w641 w643] -> w626
                  frame #0 {
                  }
                  frame #1 {
                  }
                }
                n172 = Compound Arithmetic op=OR("UPDT COM 9", w620, w613, w612, w611) -> (w621:bool)
                n173 = Compound Arithmetic op=OR(w613, w612, w611) -> (w610:bool)
              }
            }
          }
          n174 = VISA Flush I/O Buffer(VISA resource name=w561, error in (no error)=w562) -> (VISA resource name out=w564:refnum<visa-resource-name>, error out=w563:errorcluster)  [unwired: 1 in]
          n175 = VISA Close(VISA resource name=w564, error in (no error)=w563) -> (error out=w565:errorcluster)
        }
        n176 = Close File(refnum=w555, error in=w554) -> (path=w548:path, error out=w549:errorcluster)
        n177 = Strip Path(path=w548) -> (stripped path=w551:path)  [unwired: 1 out]
        n178 = Concatenate Strings(w546, string ? ("string")) -> (w544:string)
        n179 = Build Path(base path=w551, name or relative path=w544) -> (appended path=w552:path)
        n180 = Copy(8:w549, 10:w552, 11:w548) -> (0:w550:errorcluster)  [unwired: 2 in, 2 out]
        n181 = Delete(path (use dialog)=w548, error in=w550) -> (error out=w547:errorcluster)  [unwired: 3 in, 2 out]
      }
    }
  }
  n182 = while {
    tunnel: [w648] -> w25
    tunnel: [w666] -> w26
    tunnel: w53 -> [w649]
    stop <- w647 stop-if-true
    w665 = bool ?
    n183 = Obtain Notifier(name (unnamed)=string ?, notification data type=w665, create if not found? (T)=w665, error in (no error)=w649) -> (notifier out=w662:refnum<notifier>, error out=w663:errorcluster)  [unwired: 1 out]
    n184 = Obtain Notifier(name (unnamed)=string ?, notification data type=path ?, create if not found? (T)=bool ?) -> (notifier out=w658:refnum<notifier>, error out=w659:errorcluster)  [unwired: 1 in, 1 out]
    n185 = Obtain Notifier(name (unnamed)=string ?, notification data type=u32 ?, create if not found? (T)=bool ?) -> (notifier out=w652:refnum<notifier>, error out=w653:errorcluster)  [unwired: 1 in, 1 out]
    n186 = Get Notifier Status(notifier=w662, error in (no error)=w663) -> (current notification=w647:bool)  [unwired: 4 out]
    n187 = Get Notifier Status(notifier=w658, error in (no error)=w659) -> (current notification=w657:path)  [unwired: 4 out]
    n188 = Get Notifier Status(notifier=w652, error in (no error)=w653) -> (current notification=w651:u32)  [unwired: 4 out]
    n189 = Compound Arithmetic op=AND(invert w647, "Use RCVR 5") -> (w645:bool)
    n190 = case shown="True" w645 {
      tunnel: w651 -> [_ w669]
      tunnel: [w667 w685] -> w666
      tunnel: w657 -> [_ w670]
      tunnel: [w667 w679] -> w648
      frame #0 {
        w667 = errorcluster ? ("error in (no error)")
        n191 = Wait (ms)(milliseconds to wait=u32 ?) -> ()  [unwired: 1 out]
      }
      frame #1 {
        n192 = call "create RCVR files.vi"("Sample rate in"=w669, "Save Path"=w670, "Name of RCVR 1"="Name of RCVR 5") -> ("sample rate out"=w672:u32, "error out"=w673:errorcluster, "refnum out"=w674:refnum<file>, "Name of file out"=w675:string)  [unwired: 5 in]
        n193 = while {
          tunnel: [w701] -> w687
          tunnel: [w693] -> w686
          tunnel: [w699] -> w685
          shift-right: [w691] -> w678
          shift-left: w675 -> [w691]
          tunnel: w674 -> [w690]
          tunnel: w673 -> [w689]
          tunnel: w672 -> [w688]
          stop <- w692 stop-if-true
          n194 = Unbundle By Name("COM Port 5") -> ("COM Port"=w706:refnum<visa-resource-name>, "baud rate"=w705:u32, "data bits"=w704:u16, "parity"=w703:enum16{"None", "Odd", "Even", "Mark", "Space"}, "flow control"=w702:u16)
          n195 = call-poly "VISA Configure Serial Port"("VISA resource name"=w706, "timeout (10sec)"=u32 ?, "baud rate (9600)"=w705, "data bits (8)"=w704, "parity (0:none)"=w703, "error in (no error)"=errorcluster ?, "flow control (0:none)"=w702) -> ("VISA resource name out"=w709:refnum<visa-resource-name>, "error out"=w708:errorcluster)  [unwired: 7 in]
          n196 = while {
            tunnel: [w721] -> w695
            tunnel: w709 -> [w720]
            tunnel: [w718] -> w701
            shift-right: [w717] -> w696
            shift-left: w708 -> [w719]
            tunnel: [w716] -> w693
            tunnel: [w713] -> w692
            tunnel: w690 -> [w712]
            tunnel: w689 -> [w711]
            tunnel: w688 -> [w710]
            stop <- w714 stop-if-true
            n197 = call "Elapsed Time5"("Time Target (s)"=w710) -> ("Time has Elapsed"=w715:bool)  [unwired: 11 in, 7 out]
            n198 = case shown="False" w715 {
              tunnel: [w732 w736] -> w721
              tunnel: w720 -> [w732 w768]
              tunnel: w719 -> [w731 w767]
              tunnel: [w723 w762] -> w718
              tunnel: [w731 w760] -> w717
              tunnel: [w727 w755] -> w714
              tunnel: [w722 w752] -> w716
              tunnel: [bool ? w744] -> w713
              tunnel: w712 -> [w723 w734]
              tunnel: w711 -> [w722 w733]
              frame #0 {
                w726 = bool ?
                n199 = Obtain Notifier(name (unnamed)=string ?, notification data type=w726, create if not found? (T)=w726) -> (notifier out=w730:refnum<notifier>, error out=w729:errorcluster)  [unwired: 1 in, 1 out]
                n200 = Get Notifier Status(notifier=w730, error in (no error)=w729) -> (current notification=w727:bool)  [unwired: 4 out]
                n201 = Wait (ms)(milliseconds to wait=u32 ?) -> ()  [unwired: 1 out]
              }
              frame #1 {
                w737 = T3 ? items=["Flush Receive Buffer", "Write Transmit Buffer to Device", "Flush Receive Buffer (No I/O)", "Flush Transmit Buffer"] ("Mask")
                w738 = T3 ? items=["Flush Receive Buffer", "Write Transmit Buffer to Device", "Flush Receive Buffer (No I/O)", "Flush Transmit Buffer"] ("Mask")
                w743 = bool ?
                w756 = bool ?
                n202 = property class="Instr"(reference=w768, error in=w767) -> (reference out=w766:refnum<visa-resource-name>, error out=w765:errorcluster, "Bytes at Port"=w764:u32)
                n203 = Obtain Notifier(name (unnamed)=string ?, notification data type=w743, create if not found? (T)=w743) -> (notifier out=w749:refnum<notifier>, error out=w748:errorcluster)  [unwired: 1 in, 1 out]
                n204 = VISA Read(VISA resource name=w766, byte count=w764, error in (no error)=w765) -> (VISA resource name out=w742:refnum<visa-resource-name>, read buffer=w763:string, error out=w741:errorcluster)  [unwired: 1 out]
                n205 = Get Notifier Status(notifier=w749, error in (no error)=w748) -> (current notification=w745:bool)  [unwired: 4 out]
                n206 = call "RTK last 10 nema returns.vi"("x"=w763) -> ("Array"=→"Last 10 RCVR 5":string[])  [unwired: 10 in]
                n207 = VISA Flush I/O Buffer(VISA resource name=w742, mask (16)=w738, error in (no error)=w741) -> (VISA resource name out=w739:refnum<visa-resource-name>, error out=w740:errorcluster)
                n208 = Write to Text File(file (use dialog)=w734, text=w763, error in=w733) -> (refnum out=w762:refnum<file>, error out=w753:errorcluster)  [unwired: 1 in, 1 out]
                n209 = VISA Flush I/O Buffer(VISA resource name=w739, mask (16)=w737, error in (no error)=w740) -> (VISA resource name out=w736:refnum<visa-resource-name>, error out=w735:errorcluster)
                n210 = case shown="No Error" w753 {
                  selector: w753 -> [w769 w771]
                  tunnel: [bool ? bool ?] -> w746
                  tunnel: [w769 w771] -> w752
                  frame #0 {
                  }
                  frame #1 {
                  }
                }
                n211 = Obtain Notifier(name (unnamed)=string ?, notification data type=w756, create if not found? (T)=w756) -> (notifier out=w759:refnum<notifier>, error out=w758:errorcluster)  [unwired: 1 in, 1 out]
                n212 = Get Notifier Status(notifier=w759, error in (no error)=w758) -> (current notification=w747:bool)  [unwired: 4 out]
                n213 = case shown="No Error" w735 {
                  selector: w735 -> [w773 w775]
                  tunnel: [bool ? bool ?] -> w754
                  tunnel: [w773 w775] -> w760
                  frame #0 {
                  }
                  frame #1 {
                  }
                }
                n214 = Compound Arithmetic op=OR("UPDT COM 5", w754, w747, w746, w745) -> (w755:bool)
                n215 = Compound Arithmetic op=OR(w747, w746, w745) -> (w744:bool)
              }
            }
          }
          n216 = VISA Flush I/O Buffer(VISA resource name=w695, error in (no error)=w696) -> (VISA resource name out=w698:refnum<visa-resource-name>, error out=w697:errorcluster)  [unwired: 1 in]
          n217 = VISA Close(VISA resource name=w698, error in (no error)=w697) -> (error out=w699:errorcluster)
        }
        n218 = Close File(refnum=w687, error in=w686) -> (path=w680:path, error out=w681:errorcluster)
        n219 = Strip Path(path=w680) -> (stripped path=w683:path)  [unwired: 1 out]
        n220 = Concatenate Strings(w678, string ? ("string")) -> (w676:string)
        n221 = Build Path(base path=w683, name or relative path=w676) -> (appended path=w684:path)
        n222 = Copy(8:w681, 10:w684, 11:w680) -> (0:w682:errorcluster)  [unwired: 2 in, 2 out]
        n223 = Delete(path (use dialog)=w680, error in=w682) -> (error out=w679:errorcluster)  [unwired: 3 in, 2 out]
      }
    }
  }
  n224 = while {
    tunnel: [w780] -> w51
    tunnel: [w798] -> w52
    tunnel: w53 -> [w781]
    stop <- w779 stop-if-true
    w797 = bool ?
    n225 = Obtain Notifier(name (unnamed)=string ?, notification data type=w797, create if not found? (T)=w797, error in (no error)=w781) -> (notifier out=w794:refnum<notifier>, error out=w795:errorcluster)  [unwired: 1 out]
    n226 = Obtain Notifier(name (unnamed)=string ?, notification data type=path ?, create if not found? (T)=bool ?) -> (notifier out=w790:refnum<notifier>, error out=w791:errorcluster)  [unwired: 1 in, 1 out]
    n227 = Obtain Notifier(name (unnamed)=string ?, notification data type=u32 ?, create if not found? (T)=bool ?) -> (notifier out=w784:refnum<notifier>, error out=w785:errorcluster)  [unwired: 1 in, 1 out]
    n228 = Get Notifier Status(notifier=w794, error in (no error)=w795) -> (current notification=w779:bool)  [unwired: 4 out]
    n229 = Get Notifier Status(notifier=w790, error in (no error)=w791) -> (current notification=w789:path)  [unwired: 4 out]
    n230 = Get Notifier Status(notifier=w784, error in (no error)=w785) -> (current notification=w783:u32)  [unwired: 4 out]
    n231 = Compound Arithmetic op=AND(invert w779, "Use RCVR 10") -> (w777:bool)
    n232 = case shown="True" w777 {
      tunnel: w783 -> [_ w801]
      tunnel: [w799 w817] -> w798
      tunnel: w789 -> [_ w802]
      tunnel: [w799 w811] -> w780
      frame #0 {
        w799 = errorcluster ? ("error in (no error)")
        n233 = Wait (ms)(milliseconds to wait=u32 ?) -> ()  [unwired: 1 out]
      }
      frame #1 {
        n234 = call "create RCVR files.vi"("Sample rate in"=w801, "Save Path"=w802, "Name of RCVR 1"="Name of RCVR 10") -> ("sample rate out"=w804:u32, "error out"=w805:errorcluster, "refnum out"=w806:refnum<file>, "Name of file out"=w807:string)  [unwired: 5 in]
        n235 = while {
          tunnel: w806 -> [w841]
          tunnel: w805 -> [w840]
          tunnel: [w831] -> w819
          tunnel: [w822] -> w818
          tunnel: [w829] -> w817
          tunnel: w804 -> [w824]
          shift-right: [w820] -> w810
          shift-left: w807 -> [w820]
          stop <- w821 stop-if-true
          n236 = Unbundle By Name("COM Port 10") -> ("COM Port"=w836:refnum<visa-resource-name>, "baud rate"=w835:u32, "data bits"=w834:u16, "parity"=w833:enum16{"None", "Odd", "Even", "Mark", "Space"}, "flow control"=w832:u16)
          n237 = call-poly "VISA Configure Serial Port"("VISA resource name"=w836, "timeout (10sec)"=u32 ?, "baud rate (9600)"=w835, "data bits (8)"=w834, "parity (0:none)"=w833, "error in (no error)"=errorcluster ?, "flow control (0:none)"=w832) -> ("VISA resource name out"=w839:refnum<visa-resource-name>, "error out"=w838:errorcluster)  [unwired: 7 in]
          n238 = while {
            tunnel: [w853] -> w825
            tunnel: w841 -> [w850]
            tunnel: w840 -> [w848]
            tunnel: w839 -> [w852]
            tunnel: [w849] -> w831
            tunnel: w824 -> [w845]
            shift-right: [w847] -> w826
            shift-left: w838 -> [w851]
            tunnel: [w846] -> w822
            tunnel: [w842] -> w821
            stop <- w843 stop-if-true
            n239 = call "Elapsed Time10"("Time Target (s)"=w845) -> ("Time has Elapsed"=w844:bool)  [unwired: 11 in, 7 out]
            n240 = case shown="True" w844 {
              tunnel: [w864 w866] -> w853
              tunnel: w852 -> [w864 w900]
              tunnel: w851 -> [w863 w899]
              tunnel: w850 -> [w862 w894]
              tunnel: [w862 w893] -> w849
              tunnel: w848 -> [w861 w892]
              tunnel: [w863 w890] -> w847
              tunnel: [w857 w885] -> w843
              tunnel: [w861 w882] -> w846
              tunnel: [bool ? w874] -> w842
              frame #0 {
                w856 = bool ?
                n241 = Obtain Notifier(name (unnamed)=string ?, notification data type=w856, create if not found? (T)=w856) -> (notifier out=w860:refnum<notifier>, error out=w859:errorcluster)  [unwired: 1 in, 1 out]
                n242 = Get Notifier Status(notifier=w860, error in (no error)=w859) -> (current notification=w857:bool)  [unwired: 4 out]
                n243 = Wait (ms)(milliseconds to wait=u32 ?) -> ()  [unwired: 1 out]
              }
              frame #1 {
                w867 = T3 ? items=["Flush Receive Buffer", "Write Transmit Buffer to Device", "Flush Receive Buffer (No I/O)", "Flush Transmit Buffer"] ("Mask")
                w868 = T3 ? items=["Flush Receive Buffer", "Write Transmit Buffer to Device", "Flush Receive Buffer (No I/O)", "Flush Transmit Buffer"] ("Mask")
                w873 = bool ?
                w886 = bool ?
                n244 = property class="Instr"(reference=w900, error in=w899) -> (reference out=w898:refnum<visa-resource-name>, error out=w897:errorcluster, "Bytes at Port"=w896:u32)
                n245 = Obtain Notifier(name (unnamed)=string ?, notification data type=w873, create if not found? (T)=w873) -> (notifier out=w879:refnum<notifier>, error out=w878:errorcluster)  [unwired: 1 in, 1 out]
                n246 = VISA Read(VISA resource name=w898, byte count=w896, error in (no error)=w897) -> (VISA resource name out=w872:refnum<visa-resource-name>, read buffer=w895:string, error out=w871:errorcluster)  [unwired: 1 out]
                n247 = Get Notifier Status(notifier=w879, error in (no error)=w878) -> (current notification=w875:bool)  [unwired: 4 out]
                n248 = call "RTK last 10 nema returns.vi"("x"=w895) -> ("Array"=→"Last 10 RCVR 10":string[])  [unwired: 10 in]
                n249 = VISA Flush I/O Buffer(VISA resource name=w872, mask (16)=w868, error in (no error)=w871) -> (VISA resource name out=w869:refnum<visa-resource-name>, error out=w870:errorcluster)
                n250 = Write to Text File(file (use dialog)=w894, text=w895, error in=w892) -> (refnum out=w893:refnum<file>, error out=w883:errorcluster)  [unwired: 1 in, 1 out]
                n251 = VISA Flush I/O Buffer(VISA resource name=w869, mask (16)=w867, error in (no error)=w870) -> (VISA resource name out=w866:refnum<visa-resource-name>, error out=w865:errorcluster)
                n252 = case shown="No Error" w883 {
                  selector: w883 -> [w901 w903]
                  tunnel: [bool ? bool ?] -> w876
                  tunnel: [w901 w903] -> w882
                  frame #0 {
                  }
                  frame #1 {
                  }
                }
                n253 = Obtain Notifier(name (unnamed)=string ?, notification data type=w886, create if not found? (T)=w886) -> (notifier out=w889:refnum<notifier>, error out=w888:errorcluster)  [unwired: 1 in, 1 out]
                n254 = Get Notifier Status(notifier=w889, error in (no error)=w888) -> (current notification=w877:bool)  [unwired: 4 out]
                n255 = case shown="No Error" w865 {
                  selector: w865 -> [w905 w907]
                  tunnel: [bool ? bool ?] -> w884
                  tunnel: [w905 w907] -> w890
                  frame #0 {
                  }
                  frame #1 {
                  }
                }
                n256 = Compound Arithmetic op=OR("UPDT COM 10", w884, w877, w876, w875) -> (w885:bool)
                n257 = Compound Arithmetic op=OR(w877, w876, w875) -> (w874:bool)
              }
            }
          }
          n258 = VISA Flush I/O Buffer(VISA resource name=w825, error in (no error)=w826) -> (VISA resource name out=w828:refnum<visa-resource-name>, error out=w827:errorcluster)  [unwired: 1 in]
          n259 = VISA Close(VISA resource name=w828, error in (no error)=w827) -> (error out=w829:errorcluster)
        }
        n260 = Close File(refnum=w819, error in=w818) -> (path=w812:path, error out=w813:errorcluster)
        n261 = Strip Path(path=w812) -> (stripped path=w815:path)  [unwired: 1 out]
        n262 = Concatenate Strings(w810, string ? ("string")) -> (w808:string)
        n263 = Build Path(base path=w815, name or relative path=w808) -> (appended path=w816:path)
        n264 = Copy(8:w813, 10:w816, 11:w812) -> (0:w814:errorcluster)  [unwired: 2 in, 2 out]
        n265 = Delete(path (use dialog)=w812, error in=w814) -> (error out=w811:errorcluster)  [unwired: 3 in, 2 out]
      }
    }
  }
  n266 = while {
    tunnel: [w912] -> w27
    tunnel: [w930] -> w28
    tunnel: w53 -> [w913]
    stop <- w911 stop-if-true
    w929 = bool ?
    n267 = Obtain Notifier(name (unnamed)=string ?, notification data type=w929, create if not found? (T)=w929, error in (no error)=w913) -> (notifier out=w926:refnum<notifier>, error out=w927:errorcluster)  [unwired: 1 out]
    n268 = Obtain Notifier(name (unnamed)=string ?, notification data type=path ?, create if not found? (T)=bool ?) -> (notifier out=w922:refnum<notifier>, error out=w923:errorcluster)  [unwired: 1 in, 1 out]
    n269 = Obtain Notifier(name (unnamed)=string ?, notification data type=u32 ?, create if not found? (T)=bool ?) -> (notifier out=w916:refnum<notifier>, error out=w917:errorcluster)  [unwired: 1 in, 1 out]
    n270 = Get Notifier Status(notifier=w926, error in (no error)=w927) -> (current notification=w911:bool)  [unwired: 4 out]
    n271 = Get Notifier Status(notifier=w922, error in (no error)=w923) -> (current notification=w921:path)  [unwired: 4 out]
    n272 = Get Notifier Status(notifier=w916, error in (no error)=w917) -> (current notification=w915:u32)  [unwired: 4 out]
    n273 = Compound Arithmetic op=AND(invert w911, "Use RCVR 4") -> (w909:bool)
    n274 = case shown="True" w909 {
      tunnel: w915 -> [_ w933]
      tunnel: [w931 w949] -> w930
      tunnel: w921 -> [_ w934]
      tunnel: [w931 w943] -> w912
      frame #0 {
        w931 = errorcluster ? ("error in (no error)")
        n275 = Wait (ms)(milliseconds to wait=u32 ?) -> ()  [unwired: 1 out]
      }
      frame #1 {
        n276 = call "create RCVR files.vi"("Sample rate in"=w933, "Save Path"=w934, "Name of RCVR 1"="Name of RCVR 4") -> ("sample rate out"=w936:u32, "error out"=w937:errorcluster, "refnum out"=w938:refnum<file>, "Name of file out"=w939:string)  [unwired: 5 in]
        n277 = while {
          tunnel: w938 -> [w973]
          tunnel: w937 -> [w972]
          tunnel: [w963] -> w951
          tunnel: [w954] -> w950
          tunnel: [w961] -> w949
          tunnel: w936 -> [w956]
          shift-right: [w952] -> w942
          shift-left: w939 -> [w952]
          stop <- w953 stop-if-true
          n278 = Unbundle By Name("COM Port 4") -> ("COM Port"=w968:refnum<visa-resource-name>, "baud rate"=w967:u32, "data bits"=w966:u16, "parity"=w965:enum16{"None", "Odd", "Even", "Mark", "Space"}, "flow control"=w964:u16)
          n279 = call-poly "VISA Configure Serial Port"("VISA resource name"=w968, "timeout (10sec)"=u32 ?, "baud rate (9600)"=w967, "data bits (8)"=w966, "parity (0:none)"=w965, "error in (no error)"=errorcluster ?, "flow control (0:none)"=w964) -> ("VISA resource name out"=w971:refnum<visa-resource-name>, "error out"=w970:errorcluster)  [unwired: 7 in]
          n280 = while {
            tunnel: [w985] -> w957
            tunnel: w973 -> [w982]
            tunnel: w972 -> [w980]
            tunnel: w971 -> [w984]
            tunnel: [w981] -> w963
            tunnel: w956 -> [w977]
            shift-right: [w979] -> w958
            shift-left: w970 -> [w983]
            tunnel: [w978] -> w954
            tunnel: [w974] -> w953
            stop <- w975 stop-if-true
            n281 = call "Elapsed Time4"("Time Target (s)"=w977) -> ("Time has Elapsed"=w976:bool)  [unwired: 11 in, 7 out]
            n282 = case shown="False" w976 {
              tunnel: [w996 w998] -> w985
              tunnel: w984 -> [w996 w1032]
              tunnel: w983 -> [w995 w1031]
              tunnel: w982 -> [w994 w1026]
              tunnel: [w994 w1025] -> w981
              tunnel: w980 -> [w993 w1024]
              tunnel: [w995 w1022] -> w979
              tunnel: [w989 w1017] -> w975
              tunnel: [w993 w1014] -> w978
              tunnel: [bool ? w1006] -> w974
              frame #0 {
                w988 = bool ?
                n283 = Obtain Notifier(name (unnamed)=string ?, notification data type=w988, create if not found? (T)=w988) -> (notifier out=w992:refnum<notifier>, error out=w991:errorcluster)  [unwired: 1 in, 1 out]
                n284 = Get Notifier Status(notifier=w992, error in (no error)=w991) -> (current notification=w989:bool)  [unwired: 4 out]
                n285 = Wait (ms)(milliseconds to wait=u32 ?) -> ()  [unwired: 1 out]
              }
              frame #1 {
                w999 = T3 ? items=["Flush Receive Buffer", "Write Transmit Buffer to Device", "Flush Receive Buffer (No I/O)", "Flush Transmit Buffer"] ("Mask")
                w1000 = T3 ? items=["Flush Receive Buffer", "Write Transmit Buffer to Device", "Flush Receive Buffer (No I/O)", "Flush Transmit Buffer"] ("Mask")
                w1005 = bool ?
                w1018 = bool ?
                n286 = property class="Instr"(reference=w1032, error in=w1031) -> (reference out=w1030:refnum<visa-resource-name>, error out=w1029:errorcluster, "Bytes at Port"=w1028:u32)
                n287 = Obtain Notifier(name (unnamed)=string ?, notification data type=w1005, create if not found? (T)=w1005) -> (notifier out=w1011:refnum<notifier>, error out=w1010:errorcluster)  [unwired: 1 in, 1 out]
                n288 = VISA Read(VISA resource name=w1030, byte count=w1028, error in (no error)=w1029) -> (VISA resource name out=w1004:refnum<visa-resource-name>, read buffer=w1027:string, error out=w1003:errorcluster)  [unwired: 1 out]
                n289 = Get Notifier Status(notifier=w1011, error in (no error)=w1010) -> (current notification=w1007:bool)  [unwired: 4 out]
                n290 = call "RTK last 10 nema returns.vi"("x"=w1027) -> ("Array"=→"Last 10 RCVR 4":string[])  [unwired: 10 in]
                n291 = VISA Flush I/O Buffer(VISA resource name=w1004, mask (16)=w1000, error in (no error)=w1003) -> (VISA resource name out=w1001:refnum<visa-resource-name>, error out=w1002:errorcluster)
                n292 = Write to Text File(file (use dialog)=w1026, text=w1027, error in=w1024) -> (refnum out=w1025:refnum<file>, error out=w1015:errorcluster)  [unwired: 1 in, 1 out]
                n293 = VISA Flush I/O Buffer(VISA resource name=w1001, mask (16)=w999, error in (no error)=w1002) -> (VISA resource name out=w998:refnum<visa-resource-name>, error out=w997:errorcluster)
                n294 = case shown="No Error" w1015 {
                  selector: w1015 -> [w1033 w1035]
                  tunnel: [bool ? bool ?] -> w1008
                  tunnel: [w1033 w1035] -> w1014
                  frame #0 {
                  }
                  frame #1 {
                  }
                }
                n295 = Obtain Notifier(name (unnamed)=string ?, notification data type=w1018, create if not found? (T)=w1018) -> (notifier out=w1021:refnum<notifier>, error out=w1020:errorcluster)  [unwired: 1 in, 1 out]
                n296 = Get Notifier Status(notifier=w1021, error in (no error)=w1020) -> (current notification=w1009:bool)  [unwired: 4 out]
                n297 = case shown="No Error" w997 {
                  selector: w997 -> [w1037 w1039]
                  tunnel: [bool ? bool ?] -> w1016
                  tunnel: [w1037 w1039] -> w1022
                  frame #0 {
                  }
                  frame #1 {
                  }
                }
                n298 = Compound Arithmetic op=OR("UPDT COM 4", w1016, w1009, w1008, w1007) -> (w1017:bool)
                n299 = Compound Arithmetic op=OR(w1009, w1008, w1007) -> (w1006:bool)
              }
            }
          }
          n300 = VISA Flush I/O Buffer(VISA resource name=w957, error in (no error)=w958) -> (VISA resource name out=w960:refnum<visa-resource-name>, error out=w959:errorcluster)  [unwired: 1 in]
          n301 = VISA Close(VISA resource name=w960, error in (no error)=w959) -> (error out=w961:errorcluster)
        }
        n302 = Close File(refnum=w951, error in=w950) -> (path=w944:path, error out=w945:errorcluster)
        n303 = Strip Path(path=w944) -> (stripped path=w947:path)  [unwired: 1 out]
        n304 = Concatenate Strings(w942, string ? ("string")) -> (w940:string)
        n305 = Build Path(base path=w947, name or relative path=w940) -> (appended path=w948:path)
        n306 = Copy(8:w945, 10:w948, 11:w944) -> (0:w946:errorcluster)  [unwired: 2 in, 2 out]
        n307 = Delete(path (use dialog)=w944, error in=w946) -> (error out=w943:errorcluster)  [unwired: 3 in, 2 out]
      }
    }
  }
  n308 = while {
    tunnel: [w1044] -> w29
    tunnel: [w1062] -> w30
    tunnel: w53 -> [w1045]
    stop <- w1043 stop-if-true
    w1061 = bool ?
    n309 = Obtain Notifier(name (unnamed)=string ?, notification data type=w1061, create if not found? (T)=w1061, error in (no error)=w1045) -> (notifier out=w1058:refnum<notifier>, error out=w1059:errorcluster)  [unwired: 1 out]
    n310 = Obtain Notifier(name (unnamed)=string ?, notification data type=path ?, create if not found? (T)=bool ?) -> (notifier out=w1054:refnum<notifier>, error out=w1055:errorcluster)  [unwired: 1 in, 1 out]
    n311 = Obtain Notifier(name (unnamed)=string ?, notification data type=u32 ?, create if not found? (T)=bool ?) -> (notifier out=w1048:refnum<notifier>, error out=w1049:errorcluster)  [unwired: 1 in, 1 out]
    n312 = Get Notifier Status(notifier=w1058, error in (no error)=w1059) -> (current notification=w1043:bool)  [unwired: 4 out]
    n313 = Get Notifier Status(notifier=w1054, error in (no error)=w1055) -> (current notification=w1053:path)  [unwired: 4 out]
    n314 = Get Notifier Status(notifier=w1048, error in (no error)=w1049) -> (current notification=w1047:u32)  [unwired: 4 out]
    n315 = Compound Arithmetic op=AND(invert w1043, "Use RCVR 3") -> (w1041:bool)
    n316 = case shown="True" w1041 {
      tunnel: w1047 -> [_ w1065]
      tunnel: [w1063 w1081] -> w1062
      tunnel: w1053 -> [_ w1067]
      tunnel: [w1063 w1075] -> w1044
      frame #0 {
        w1063 = errorcluster ? ("error in (no error)")
        n317 = Wait (ms)(milliseconds to wait=u32 ?) -> ()  [unwired: 1 out]
      }
      frame #1 {
        n318 = call "create RCVR files.vi"("Sample rate in"=w1065, "Save Path"=w1067, "Name of RCVR 1"="Name of RCVR 3") -> ("sample rate out"=w1068:u32, "error out"=w1069:errorcluster, "refnum out"=w1070:refnum<file>, "Name of file out"=w1071:string)  [unwired: 5 in]
        n319 = while {
          tunnel: w1070 -> [w1105]
          tunnel: w1069 -> [w1104]
          tunnel: [w1095] -> w1083
          tunnel: [w1086] -> w1082
          tunnel: [w1093] -> w1081
          tunnel: w1068 -> [w1088]
          shift-right: [w1084] -> w1074
          shift-left: w1071 -> [w1084]
          stop <- w1085 stop-if-true
          n320 = Unbundle By Name("COM Port 3") -> ("COM Port"=w1100:refnum<visa-resource-name>, "baud rate"=w1099:u32, "data bits"=w1098:u16, "parity"=w1097:enum16{"None", "Odd", "Even", "Mark", "Space"}, "flow control"=w1096:u16)
          n321 = call-poly "VISA Configure Serial Port"("VISA resource name"=w1100, "timeout (10sec)"=u32 ?, "baud rate (9600)"=w1099, "data bits (8)"=w1098, "parity (0:none)"=w1097, "error in (no error)"=errorcluster ?, "flow control (0:none)"=w1096) -> ("VISA resource name out"=w1103:refnum<visa-resource-name>, "error out"=w1102:errorcluster)  [unwired: 7 in]
          n322 = while {
            tunnel: [w1117] -> w1089
            tunnel: w1105 -> [w1114]
            tunnel: w1104 -> [w1112]
            tunnel: w1103 -> [w1116]
            tunnel: [w1113] -> w1095
            tunnel: w1088 -> [w1109]
            shift-right: [w1111] -> w1090
            shift-left: w1102 -> [w1115]
            tunnel: [w1110] -> w1086
            tunnel: [w1106] -> w1085
            stop <- w1107 stop-if-true
            n323 = call "Elapsed Time3"("Time Target (s)"=w1109) -> ("Time has Elapsed"=w1108:bool)  [unwired: 11 in, 7 out]
            n324 = case shown="True" w1108 {
              tunnel: [w1128 w1130] -> w1117
              tunnel: w1116 -> [w1128 w1164]
              tunnel: w1115 -> [w1127 w1163]
              tunnel: w1114 -> [w1126 w1158]
              tunnel: [w1126 w1157] -> w1113
              tunnel: w1112 -> [w1125 w1156]
              tunnel: [w1127 w1154] -> w1111
              tunnel: [w1121 w1149] -> w1107
              tunnel: [w1125 w1146] -> w1110
              tunnel: [bool ? w1138] -> w1106
              frame #0 {
                w1120 = bool ?
                n325 = Obtain Notifier(name (unnamed)=string ?, notification data type=w1120, create if not found? (T)=w1120) -> (notifier out=w1124:refnum<notifier>, error out=w1123:errorcluster)  [unwired: 1 in, 1 out]
                n326 = Get Notifier Status(notifier=w1124, error in (no error)=w1123) -> (current notification=w1121:bool)  [unwired: 4 out]
                n327 = Wait (ms)(milliseconds to wait=u32 ?) -> ()  [unwired: 1 out]
              }
              frame #1 {
                w1131 = T3 ? items=["Flush Receive Buffer", "Write Transmit Buffer to Device", "Flush Receive Buffer (No I/O)", "Flush Transmit Buffer"] ("Mask")
                w1132 = T3 ? items=["Flush Receive Buffer", "Write Transmit Buffer to Device", "Flush Receive Buffer (No I/O)", "Flush Transmit Buffer"] ("Mask")
                w1137 = bool ?
                w1150 = bool ?
                n328 = property class="Instr"(reference=w1164, error in=w1163) -> (reference out=w1162:refnum<visa-resource-name>, error out=w1161:errorcluster, "Bytes at Port"=w1160:u32)
                n329 = Obtain Notifier(name (unnamed)=string ?, notification data type=w1137, create if not found? (T)=w1137) -> (notifier out=w1143:refnum<notifier>, error out=w1142:errorcluster)  [unwired: 1 in, 1 out]
                n330 = VISA Read(VISA resource name=w1162, byte count=w1160, error in (no error)=w1161) -> (VISA resource name out=w1136:refnum<visa-resource-name>, read buffer=w1159:string, error out=w1135:errorcluster)  [unwired: 1 out]
                n331 = Get Notifier Status(notifier=w1143, error in (no error)=w1142) -> (current notification=w1139:bool)  [unwired: 4 out]
                n332 = call "RTK last 10 nema returns.vi"("x"=w1159) -> ("Array"=→"Last 10 RCVR 3":string[])  [unwired: 10 in]
                n333 = VISA Flush I/O Buffer(VISA resource name=w1136, mask (16)=w1132, error in (no error)=w1135) -> (VISA resource name out=w1133:refnum<visa-resource-name>, error out=w1134:errorcluster)
                n334 = Write to Text File(file (use dialog)=w1158, text=w1159, error in=w1156) -> (refnum out=w1157:refnum<file>, error out=w1147:errorcluster)  [unwired: 1 in, 1 out]
                n335 = VISA Flush I/O Buffer(VISA resource name=w1133, mask (16)=w1131, error in (no error)=w1134) -> (VISA resource name out=w1130:refnum<visa-resource-name>, error out=w1129:errorcluster)
                n336 = case shown="No Error" w1147 {
                  selector: w1147 -> [w1165 w1167]
                  tunnel: [bool ? bool ?] -> w1140
                  tunnel: [w1165 w1167] -> w1146
                  frame #0 {
                  }
                  frame #1 {
                  }
                }
                n337 = Obtain Notifier(name (unnamed)=string ?, notification data type=w1150, create if not found? (T)=w1150) -> (notifier out=w1153:refnum<notifier>, error out=w1152:errorcluster)  [unwired: 1 in, 1 out]
                n338 = Get Notifier Status(notifier=w1153, error in (no error)=w1152) -> (current notification=w1141:bool)  [unwired: 4 out]
                n339 = case shown="No Error" w1129 {
                  selector: w1129 -> [w1169 w1171]
                  tunnel: [bool ? bool ?] -> w1148
                  tunnel: [w1169 w1171] -> w1154
                  frame #0 {
                  }
                  frame #1 {
                  }
                }
                n340 = Compound Arithmetic op=OR("UPDT COM 3", w1148, w1141, w1140, w1139) -> (w1149:bool)
                n341 = Compound Arithmetic op=OR(w1141, w1140, w1139) -> (w1138:bool)
              }
            }
          }
          n342 = VISA Flush I/O Buffer(VISA resource name=w1089, error in (no error)=w1090) -> (VISA resource name out=w1092:refnum<visa-resource-name>, error out=w1091:errorcluster)  [unwired: 1 in]
          n343 = VISA Close(VISA resource name=w1092, error in (no error)=w1091) -> (error out=w1093:errorcluster)
        }
        n344 = Close File(refnum=w1083, error in=w1082) -> (path=w1076:path, error out=w1077:errorcluster)
        n345 = Strip Path(path=w1076) -> (stripped path=w1079:path)  [unwired: 1 out]
        n346 = Concatenate Strings(w1074, string ? ("string")) -> (w1072:string)
        n347 = Build Path(base path=w1079, name or relative path=w1072) -> (appended path=w1080:path)
        n348 = Copy(8:w1077, 10:w1080, 11:w1076) -> (0:w1078:errorcluster)  [unwired: 2 in, 2 out]
        n349 = Delete(path (use dialog)=w1076, error in=w1078) -> (error out=w1075:errorcluster)  [unwired: 3 in, 2 out]
      }
    }
  }
  n350 = while {
    tunnel: [w1176] -> w35
    tunnel: [w1194] -> w36
    tunnel: w53 -> [w1177]
    stop <- w1175 stop-if-true
    w1193 = bool ?
    n351 = Obtain Notifier(name (unnamed)=string ?, notification data type=w1193, create if not found? (T)=w1193, error in (no error)=w1177) -> (notifier out=w1190:refnum<notifier>, error out=w1191:errorcluster)  [unwired: 1 out]
    n352 = Obtain Notifier(name (unnamed)=string ?, notification data type=path ?, create if not found? (T)=bool ?) -> (notifier out=w1186:refnum<notifier>, error out=w1187:errorcluster)  [unwired: 1 in, 1 out]
    n353 = Obtain Notifier(name (unnamed)=string ?, notification data type=u32 ?, create if not found? (T)=bool ?) -> (notifier out=w1180:refnum<notifier>, error out=w1181:errorcluster)  [unwired: 1 in, 1 out]
    n354 = Get Notifier Status(notifier=w1190, error in (no error)=w1191) -> (current notification=w1175:bool)  [unwired: 4 out]
    n355 = Get Notifier Status(notifier=w1186, error in (no error)=w1187) -> (current notification=w1185:path)  [unwired: 4 out]
    n356 = Get Notifier Status(notifier=w1180, error in (no error)=w1181) -> (current notification=w1179:u32)  [unwired: 4 out]
    n357 = Compound Arithmetic op=AND(invert w1175, "Use RCVR 2") -> (w1173:bool)
    n358 = case shown="True" w1173 {
      tunnel: w1179 -> [_ w1197]
      tunnel: [w1195 w1213] -> w1194
      tunnel: w1185 -> [_ w1198]
      tunnel: [w1195 w1207] -> w1176
      frame #0 {
        w1195 = errorcluster ? ("error in (no error)")
        n359 = Wait (ms)(milliseconds to wait=u32 ?) -> ()  [unwired: 1 out]
      }
      frame #1 {
        n360 = call "create RCVR files.vi"("Sample rate in"=w1197, "Save Path"=w1198, "Name of RCVR 1"="Name of RCVR 2") -> ("sample rate out"=w1200:u32, "error out"=w1201:errorcluster, "refnum out"=w1202:refnum<file>, "Name of file out"=w1203:string)  [unwired: 5 in]
        n361 = while {
          tunnel: w1202 -> [w1237]
          tunnel: w1201 -> [w1236]
          tunnel: [w1227] -> w1215
          tunnel: [w1218] -> w1214
          tunnel: [w1225] -> w1213
          tunnel: w1200 -> [w1220]
          shift-right: [w1216] -> w1206
          shift-left: w1203 -> [w1216]
          stop <- w1217 stop-if-true
          n362 = Unbundle By Name("COM Port 2") -> ("COM Port"=w1232:refnum<visa-resource-name>, "baud rate"=w1231:u32, "data bits"=w1230:u16, "parity"=w1229:enum16{"None", "Odd", "Even", "Mark", "Space"}, "flow control"=w1228:u16)
          n363 = call-poly "VISA Configure Serial Port"("VISA resource name"=w1232, "timeout (10sec)"=u32 ?, "baud rate (9600)"=w1231, "data bits (8)"=w1230, "parity (0:none)"=w1229, "error in (no error)"=errorcluster ?, "flow control (0:none)"=w1228) -> ("VISA resource name out"=w1235:refnum<visa-resource-name>, "error out"=w1234:errorcluster)  [unwired: 7 in]
          n364 = while {
            tunnel: [w1249] -> w1221
            tunnel: w1237 -> [w1246]
            tunnel: w1236 -> [w1244]
            tunnel: w1235 -> [w1248]
            tunnel: [w1245] -> w1227
            tunnel: w1220 -> [w1241]
            shift-right: [w1243] -> w1222
            shift-left: w1234 -> [w1247]
            tunnel: [w1242] -> w1218
            tunnel: [w1238] -> w1217
            stop <- w1239 stop-if-true
            n365 = call "Elapsed Time2"("Time Target (s)"=w1241) -> ("Time has Elapsed"=w1240:bool)  [unwired: 11 in, 7 out]
            n366 = case shown="True" w1240 {
              tunnel: [w1260 w1262] -> w1249
              tunnel: w1248 -> [w1260 w1296]
              tunnel: w1247 -> [w1259 w1295]
              tunnel: w1246 -> [w1258 w1290]
              tunnel: [w1258 w1289] -> w1245
              tunnel: w1244 -> [w1257 w1288]
              tunnel: [w1259 w1286] -> w1243
              tunnel: [w1253 w1281] -> w1239
              tunnel: [w1257 w1278] -> w1242
              tunnel: [bool ? w1270] -> w1238
              frame #0 {
                w1252 = bool ?
                n367 = Obtain Notifier(name (unnamed)=string ?, notification data type=w1252, create if not found? (T)=w1252) -> (notifier out=w1256:refnum<notifier>, error out=w1255:errorcluster)  [unwired: 1 in, 1 out]
                n368 = Get Notifier Status(notifier=w1256, error in (no error)=w1255) -> (current notification=w1253:bool)  [unwired: 4 out]
                n369 = Wait (ms)(milliseconds to wait=u32 ?) -> ()  [unwired: 1 out]
              }
              frame #1 {
                w1263 = T3 ? items=["Flush Receive Buffer", "Write Transmit Buffer to Device", "Flush Receive Buffer (No I/O)", "Flush Transmit Buffer"] ("Mask")
                w1264 = T3 ? items=["Flush Receive Buffer", "Write Transmit Buffer to Device", "Flush Receive Buffer (No I/O)", "Flush Transmit Buffer"] ("Mask")
                w1269 = bool ?
                w1282 = bool ?
                n370 = property class="Instr"(reference=w1296, error in=w1295) -> (reference out=w1294:refnum<visa-resource-name>, error out=w1293:errorcluster, "Bytes at Port"=w1292:u32)
                n371 = Obtain Notifier(name (unnamed)=string ?, notification data type=w1269, create if not found? (T)=w1269) -> (notifier out=w1275:refnum<notifier>, error out=w1274:errorcluster)  [unwired: 1 in, 1 out]
                n372 = VISA Read(VISA resource name=w1294, byte count=w1292, error in (no error)=w1293) -> (VISA resource name out=w1268:refnum<visa-resource-name>, read buffer=w1291:string, error out=w1267:errorcluster)  [unwired: 1 out]
                n373 = Get Notifier Status(notifier=w1275, error in (no error)=w1274) -> (current notification=w1271:bool)  [unwired: 4 out]
                n374 = call "RTK last 10 nema returns.vi"("x"=w1291) -> ("Array"=→"Last 10 RCVR 2":string[])  [unwired: 10 in]
                n375 = VISA Flush I/O Buffer(VISA resource name=w1268, mask (16)=w1264, error in (no error)=w1267) -> (VISA resource name out=w1265:refnum<visa-resource-name>, error out=w1266:errorcluster)
                n376 = Write to Text File(file (use dialog)=w1290, text=w1291, error in=w1288) -> (refnum out=w1289:refnum<file>, error out=w1279:errorcluster)  [unwired: 1 in, 1 out]
                n377 = VISA Flush I/O Buffer(VISA resource name=w1265, mask (16)=w1263, error in (no error)=w1266) -> (VISA resource name out=w1262:refnum<visa-resource-name>, error out=w1261:errorcluster)
                n378 = case shown="No Error" w1279 {
                  selector: w1279 -> [w1297 w1299]
                  tunnel: [bool ? bool ?] -> w1272
                  tunnel: [w1297 w1299] -> w1278
                  frame #0 {
                  }
                  frame #1 {
                  }
                }
                n379 = Obtain Notifier(name (unnamed)=string ?, notification data type=w1282, create if not found? (T)=w1282) -> (notifier out=w1285:refnum<notifier>, error out=w1284:errorcluster)  [unwired: 1 in, 1 out]
                n380 = Get Notifier Status(notifier=w1285, error in (no error)=w1284) -> (current notification=w1273:bool)  [unwired: 4 out]
                n381 = case shown="No Error" w1261 {
                  selector: w1261 -> [w1301 w1303]
                  tunnel: [bool ? bool ?] -> w1280
                  tunnel: [w1301 w1303] -> w1286
                  frame #0 {
                  }
                  frame #1 {
                  }
                }
                n382 = Compound Arithmetic op=OR("UPDT COM 2", w1280, w1273, w1272, w1271) -> (w1281:bool)
                n383 = Compound Arithmetic op=OR(w1273, w1272, w1271) -> (w1270:bool)
              }
            }
          }
          n384 = VISA Flush I/O Buffer(VISA resource name=w1221, error in (no error)=w1222) -> (VISA resource name out=w1224:refnum<visa-resource-name>, error out=w1223:errorcluster)  [unwired: 1 in]
          n385 = VISA Close(VISA resource name=w1224, error in (no error)=w1223) -> (error out=w1225:errorcluster)
        }
        n386 = Close File(refnum=w1215, error in=w1214) -> (path=w1208:path, error out=w1209:errorcluster)
        n387 = Strip Path(path=w1208) -> (stripped path=w1211:path)  [unwired: 1 out]
        n388 = Concatenate Strings(w1206, string ? ("string")) -> (w1204:string)
        n389 = Build Path(base path=w1211, name or relative path=w1204) -> (appended path=w1212:path)
        n390 = Copy(8:w1209, 10:w1212, 11:w1208) -> (0:w1210:errorcluster)  [unwired: 2 in, 2 out]
        n391 = Delete(path (use dialog)=w1208, error in=w1210) -> (error out=w1207:errorcluster)  [unwired: 3 in, 2 out]
      }
    }
  }
  n392 = while {
    tunnel: [w1308] -> w37
    tunnel: [w1326] -> w38
    tunnel: w53 -> [w1309]
    stop <- w1307 stop-if-true
    w1325 = bool ?
    n393 = Obtain Notifier(name (unnamed)=string ?, notification data type=w1325, create if not found? (T)=w1325, error in (no error)=w1309) -> (notifier out=w1322:refnum<notifier>, error out=w1323:errorcluster)  [unwired: 1 out]
    n394 = Obtain Notifier(name (unnamed)=string ?, notification data type=path ?, create if not found? (T)=bool ?) -> (notifier out=w1318:refnum<notifier>, error out=w1319:errorcluster)  [unwired: 1 in, 1 out]
    n395 = Obtain Notifier(name (unnamed)=string ?, notification data type=u32 ?, create if not found? (T)=bool ?) -> (notifier out=w1312:refnum<notifier>, error out=w1313:errorcluster)  [unwired: 1 in, 1 out]
    n396 = Get Notifier Status(notifier=w1322, error in (no error)=w1323) -> (current notification=w1307:bool)  [unwired: 4 out]
    n397 = Get Notifier Status(notifier=w1318, error in (no error)=w1319) -> (current notification=w1317:path)  [unwired: 4 out]
    n398 = Get Notifier Status(notifier=w1312, error in (no error)=w1313) -> (current notification=w1311:u32)  [unwired: 4 out]
    n399 = Compound Arithmetic op=AND(invert w1307, "Use RCVR 1") -> (w1305:bool)
    n400 = case shown="True" w1305 {
      tunnel: w1311 -> [_ w1329]
      tunnel: [w1327 w1345] -> w1326
      tunnel: w1317 -> [_ w1330]
      tunnel: [w1327 w1339] -> w1308
      frame #0 {
        w1327 = errorcluster ? ("error in (no error)")
        n401 = Wait (ms)(milliseconds to wait=u32 ?) -> ()  [unwired: 1 out]
      }
      frame #1 {
        n402 = call "create RCVR files.vi"("Sample rate in"=w1329, "Save Path"=w1330, "Name of RCVR 1"="Name of RCVR 1") -> ("sample rate out"=w1332:u32, "error out"=w1333:errorcluster, "refnum out"=w1334:refnum<file>, "Name of file out"=w1335:string)  [unwired: 5 in]
        n403 = while {
          tunnel: w1334 -> [w1369]
          tunnel: w1333 -> [w1368]
          tunnel: [w1359] -> w1347
          tunnel: [w1350] -> w1346
          tunnel: [w1357] -> w1345
          tunnel: w1332 -> [w1352]
          shift-right: [w1348] -> w1338
          shift-left: w1335 -> [w1348]
          stop <- w1349 stop-if-true
          n404 = Unbundle By Name("COM Port 1") -> ("COM Port"=w1364:refnum<visa-resource-name>, "baud rate"=w1363:u32, "data bits"=w1362:u16, "parity"=w1361:enum16{"None", "Odd", "Even", "Mark", "Space"}, "flow control"=w1360:u16)
          n405 = call-poly "VISA Configure Serial Port"("VISA resource name"=w1364, "timeout (10sec)"=u32 ?, "baud rate (9600)"=w1363, "data bits (8)"=w1362, "parity (0:none)"=w1361, "error in (no error)"=errorcluster ?, "flow control (0:none)"=w1360) -> ("VISA resource name out"=w1367:refnum<visa-resource-name>, "error out"=w1366:errorcluster)  [unwired: 7 in]
          n406 = while {
            tunnel: [w1381] -> w1353
            tunnel: w1369 -> [w1378]
            tunnel: w1368 -> [w1376]
            tunnel: w1367 -> [w1380]
            tunnel: [w1377] -> w1359
            tunnel: w1352 -> [w1373]
            shift-right: [w1375] -> w1354
            shift-left: w1366 -> [w1379]
            tunnel: [w1374] -> w1350
            tunnel: [w1370] -> w1349
            stop <- w1371 stop-if-true
            n407 = call "Elapsed Time"("Time Target (s)"=w1373) -> ("Time has Elapsed"=w1372:bool)  [unwired: 11 in, 7 out]
            n408 = case shown="True" w1372 {
              tunnel: [w1392 w1394] -> w1381
              tunnel: w1380 -> [w1392 w1428]
              tunnel: w1379 -> [w1391 w1427]
              tunnel: w1378 -> [w1390 w1422]
              tunnel: [w1390 w1421] -> w1377
              tunnel: w1376 -> [w1389 w1420]
              tunnel: [w1391 w1418] -> w1375
              tunnel: [w1385 w1413] -> w1371
              tunnel: [w1389 w1410] -> w1374
              tunnel: [bool ? w1402] -> w1370
              frame #0 {
                w1384 = bool ?
                n409 = Obtain Notifier(name (unnamed)=string ?, notification data type=w1384, create if not found? (T)=w1384) -> (notifier out=w1388:refnum<notifier>, error out=w1387:errorcluster)  [unwired: 1 in, 1 out]
                n410 = Get Notifier Status(notifier=w1388, error in (no error)=w1387) -> (current notification=w1385:bool)  [unwired: 4 out]
                n411 = Wait (ms)(milliseconds to wait=u32 ?) -> ()  [unwired: 1 out]
              }
              frame #1 {
                w1395 = T3 ? items=["Flush Receive Buffer", "Write Transmit Buffer to Device", "Flush Receive Buffer (No I/O)", "Flush Transmit Buffer"] ("Mask")
                w1396 = T3 ? items=["Flush Receive Buffer", "Write Transmit Buffer to Device", "Flush Receive Buffer (No I/O)", "Flush Transmit Buffer"] ("Mask")
                w1401 = bool ?
                w1414 = bool ?
                n412 = property class="Instr"(reference=w1428, error in=w1427) -> (reference out=w1426:refnum<visa-resource-name>, error out=w1425:errorcluster, "Bytes at Port"=w1424:u32)
                n413 = Obtain Notifier(name (unnamed)=string ?, notification data type=w1401, create if not found? (T)=w1401) -> (notifier out=w1407:refnum<notifier>, error out=w1406:errorcluster)  [unwired: 1 in, 1 out]
                n414 = VISA Read(VISA resource name=w1426, byte count=w1424, error in (no error)=w1425) -> (VISA resource name out=w1400:refnum<visa-resource-name>, read buffer=w1423:string, error out=w1399:errorcluster)  [unwired: 1 out]
                n415 = Get Notifier Status(notifier=w1407, error in (no error)=w1406) -> (current notification=w1403:bool)  [unwired: 4 out]
                n416 = call "RTK last 10 nema returns.vi"("x"=w1423) -> ("Array"=→"Last 10 RCVR 1":string[])  [unwired: 10 in]
                n417 = VISA Flush I/O Buffer(VISA resource name=w1400, mask (16)=w1396, error in (no error)=w1399) -> (VISA resource name out=w1397:refnum<visa-resource-name>, error out=w1398:errorcluster)
                n418 = Write to Text File(file (use dialog)=w1422, text=w1423, error in=w1420) -> (refnum out=w1421:refnum<file>, error out=w1411:errorcluster)  [unwired: 1 in, 1 out]
                n419 = VISA Flush I/O Buffer(VISA resource name=w1397, mask (16)=w1395, error in (no error)=w1398) -> (VISA resource name out=w1394:refnum<visa-resource-name>, error out=w1393:errorcluster)
                n420 = case shown="No Error" w1411 {
                  selector: w1411 -> [w1429 w1431]
                  tunnel: [bool ? bool ?] -> w1404
                  tunnel: [w1429 w1431] -> w1410
                  frame #0 {
                  }
                  frame #1 {
                  }
                }
                n421 = Obtain Notifier(name (unnamed)=string ?, notification data type=w1414, create if not found? (T)=w1414) -> (notifier out=w1417:refnum<notifier>, error out=w1416:errorcluster)  [unwired: 1 in, 1 out]
                n422 = Get Notifier Status(notifier=w1417, error in (no error)=w1416) -> (current notification=w1405:bool)  [unwired: 4 out]
                n423 = case shown="No Error" w1393 {
                  selector: w1393 -> [w1433 w1435]
                  tunnel: [bool ? bool ?] -> w1412
                  tunnel: [w1433 w1435] -> w1418
                  frame #0 {
                  }
                  frame #1 {
                  }
                }
                n424 = Compound Arithmetic op=OR("UPDT COM 1", w1412, w1405, w1404, w1403) -> (w1413:bool)
                n425 = Compound Arithmetic op=OR(w1405, w1404, w1403) -> (w1402:bool)
              }
            }
          }
          n426 = VISA Flush I/O Buffer(VISA resource name=w1353, error in (no error)=w1354) -> (VISA resource name out=w1356:refnum<visa-resource-name>, error out=w1355:errorcluster)  [unwired: 1 in]
          n427 = VISA Close(VISA resource name=w1356, error in (no error)=w1355) -> (error out=w1357:errorcluster)
        }
        n428 = Close File(refnum=w1347, error in=w1346) -> (path=w1340:path, error out=w1341:errorcluster)
        n429 = Strip Path(path=w1340) -> (stripped path=w1343:path)  [unwired: 1 out]
        n430 = Concatenate Strings(w1338, string ? ("string")) -> (w1336:string)
        n431 = Build Path(base path=w1343, name or relative path=w1336) -> (appended path=w1344:path)
        n432 = Copy(8:w1341, 10:w1344, 11:w1340) -> (0:w1342:errorcluster)  [unwired: 2 in, 2 out]
        n433 = Delete(path (use dialog)=w1340, error in=w1342) -> (error out=w1339:errorcluster)  [unwired: 3 in, 2 out]
      }
    }
  }
  n434 = Obtain Notifier(name (unnamed)=string ?, notification data type=w78, error in (no error)=w53) -> (notifier out=w82:refnum<notifier>, error out=w80:errorcluster)  [unwired: 1 in, 1 out]
  n435 = Obtain Notifier(name (unnamed)=string ?, notification data type=w83, error in (no error)=w53) -> (notifier out=w74:refnum<notifier>, error out=w75:errorcluster)  [unwired: 1 in, 1 out]
  n436 = Send Notification(notification=w78, notifier=w82, error in (no error)=w80) -> (notifier out=w81:refnum<notifier>, error out=w79:errorcluster)
  n437 = Send Notification(notification=w73, notifier=w74, error in (no error)=w75) -> (notifier out=w77:refnum<notifier>, error out=w76:errorcluster)
  n438 = Obtain Notifier(name (unnamed)=string ?, notification data type=bool ?, error in (no error)=w53) -> (notifier out=w88:refnum<notifier>, error out=w87:errorcluster)  [unwired: 1 in, 1 out]
  n439 = Obtain Notifier(name (unnamed)=string ?, notification data type=bool ?, error in (no error)=w53) -> (notifier out=w91:refnum<notifier>, error out=w92:errorcluster)  [unwired: 1 in, 1 out]
  n440 = while {
    tunnel: w91 -> [w1465]
    tunnel: [w1438] -> w62
    tunnel: w88 -> [w1463]
    tunnel: [w1461] -> w61
    tunnel: w77 -> [w1458]
    tunnel: [w1460] -> w60
    tunnel: w81 -> [w1457]
    tunnel: [w1455] -> w59
    shift-right: [w1450] -> w66
    shift-left: w79 -> [w1456]
    shift-right: [w1448] -> w67
    shift-left: w76 -> [w1459]
    shift-right: [w1446] -> w68
    shift-left: w87 -> [w1462]
    shift-right: [w1440] -> w69
    shift-left: w92 -> [w1464]
    shift-right: [w1444] -> _
    shift-left: _ -> [w1443]
    stop <- w1437 stop-if-true
    n441 = event shown="[0] Timeout" {
      selector: _ -> [_ _ _ _]
      dyn-events: _ -> [_ _ _ _]
      timeout: i32 ? -> [_ _ _ _]
      tunnel: w1465 -> [w1500 w1548 w1557 w1593]
      tunnel: [w1500 w1547 w1560 w1593] -> w1439
      tunnel: w1464 -> [w1499 w1546 w1558 w1592]
      tunnel: [w1499 w1545 w1559 w1592] -> w1445
      tunnel: w1463 -> [w1490 w1543 w1555 w1596]
      tunnel: w1462 -> [w1489 w1544 w1556 w1595]
      tunnel: [w1487 w1544 w1556 w1577] -> w1447
      tunnel: [w1488 w1543 w1555 w1578] -> w1461
      tunnel: w1458 -> [w1494 w1540 w1552 w1588]
      tunnel: w1459 -> [w1492 w1539 w1551 w1589]
      tunnel: [w1491 w1539 w1551 w1590] -> w1449
      tunnel: [w1493 w1540 w1552 w1591] -> w1460
      tunnel: w1457 -> [w1498 w1542 w1554 w1587]
      tunnel: w1456 -> [w1485 w1541 w1553 w1586]
      tunnel: [w1496 w1541 w1553 w1585] -> w1451
      tunnel: [w1497 w1542 w1554 w1584] -> w1455
      tunnel: "Number of hours To Collect before starting new file" -> [w1484 _ _ _]
      tunnel: "Time between samples (seconds)" -> [w1486 _ _ w1574]
      tunnel: "Base File Path" -> [w1495 _ _ w1576]
      tunnel: [w1482 w1537 w1550 w1570] -> w1444
      tunnel: w1443 -> [w1481 w1537 w1550 w1570]
      tunnel: [w1480 errorcluster ? ("error out") errorcluster ? ("error out") errorcluster ? ("error out")] -> w1442
      event #0 {
        n442 = event-data() -> ()  [unwired: 1 in, 2 out]
        n443 = call "hours between scans.vi"("Number of hours To Collect before starting new file"=w1484, "Input start time"=w1481) -> ("error out"=w1480:errorcluster, "Time has Elapsed"=w1483:bool, "output next start time"=w1482:dbl)  [unwired: 7 in]
        n444 = case shown="True" w1483 {
          tunnel: w1485 -> [w1505 w1529]
          tunnel: w1498 -> [w1506 w1531]
          tunnel: [w1506 w1530] -> w1497
          tunnel: [w1505 w1528] -> w1496
          tunnel: w1495 -> [_ w1527]
          tunnel: w1494 -> [w1504 w1526]
          tunnel: [w1504 w1525] -> w1493
          tunnel: w1486 -> [_ w1524]
          tunnel: w1492 -> [w1503 w1523]
          tunnel: [w1503 w1522] -> w1491
          tunnel: w1490 -> [w1502 w1515]
          tunnel: w1489 -> [w1501 w1514]
          tunnel: [w1502 w1513] -> w1488
          tunnel: [w1501 w1512] -> w1487
          tunnel: w1486 -> [_ w1511]
          frame #0 {
          }
          frame #1 {
            n445 = Multiply(x=u32 ?, y=w1511) -> (x*y=w1509:u32)
            n446 = Send Notification(notification=bool ?, notifier=w1515, error in (no error)=w1514) -> (notifier out=w1520:refnum<notifier>, error out=w1519:errorcluster)
            n447 = Add(x=u32 ? ("milliseconds to wait"), y=w1509) -> (x+y=w1507:u32)
            n448 = while {
              tunnel: w1520 -> [w1533]
              tunnel: w1519 -> [w1534]
              tunnel: [w1534] -> w1517
              tunnel: [w1533] -> w1516
              tunnel: w1507 -> [w1532]
              stop <- bool ? ("stop 2") stop-if-true
              n449 = Wait (ms)(milliseconds to wait=w1532) -> ()  [unwired: 1 out]
            }
            n450 = Send Notification(notification=w1524, notifier=w1526, error in (no error)=w1523) -> (notifier out=w1525:refnum<notifier>, error out=w1522:errorcluster)
            n451 = Send Notification(notification=w1527, notifier=w1531, error in (no error)=w1529) -> (notifier out=w1530:refnum<notifier>, error out=w1528:errorcluster)
            n452 = Send Notification(notification=bool ?, notifier=w1516, error in (no error)=w1517) -> (notifier out=w1513:refnum<notifier>, error out=w1512:errorcluster)
          }
        }
      }
      event #1 {
        n453 = event-data() -> ()  [unwired: 1 in, 1 out]
        n454 = Send Notification(notification=bool ?, notifier=w1548, error in (no error)=w1546) -> (notifier out=w1547:refnum<notifier>, error out=w1545:errorcluster)
      }
      event #2 {
        n455 = event-data() -> ("ItemTag"=w1561:string)  [unwired: 1 in]
        n456 = case shown="\"ShutDown\"" w1561 {
          tunnel: [w1563 w1568] -> w1560
          tunnel: [w1562 w1567] -> w1559
          tunnel: w1558 -> [w1562 w1566]
          tunnel: w1557 -> [w1563 w1565]
          frame #0 {
            (unwired) bool ?
          }
          frame #1 {
            n457 = Send Notification(notification=bool ?, notifier=w1565, error in (no error)=w1566) -> (notifier out=w1568:refnum<notifier>, error out=w1567:errorcluster)
          }
        }
      }
      event #3 {
        n458 = event-data() -> ()  [unwired: 1 in, 1 out]
        n459 = Send Notification(notification=bool ?, notifier=w1596, error in (no error)=w1595) -> (notifier out=w1583:refnum<notifier>, error out=w1582:errorcluster)
        n460 = Multiply(x=u32 ?, y=w1574) -> (x*y=w1575:u32)
        n461 = Add(x=u32 ? ("milliseconds to wait"), y=w1575) -> (x+y=w1571:u32)
        n462 = Send Notification(notification=w1576, notifier=w1587, error in (no error)=w1586) -> (notifier out=w1584:refnum<notifier>, error out=w1585:errorcluster)
        n463 = Send Notification(notification=w1574, notifier=w1588, error in (no error)=w1589) -> (notifier out=w1591:refnum<notifier>, error out=w1590:errorcluster)
        n464 = while {
          tunnel: w1583 -> [w1598]
          tunnel: w1582 -> [w1599]
          tunnel: [w1599] -> w1580
          tunnel: [w1598] -> w1579
          tunnel: w1571 -> [w1597]
          stop <- bool ? ("stop 2") stop-if-true
          n465 = Wait (ms)(milliseconds to wait=w1597) -> ()  [unwired: 1 out]
        }
        n466 = Send Notification(notification=bool ?, notifier=w1579, error in (no error)=w1580) -> (notifier out=w1578:refnum<notifier>, error out=w1577:errorcluster)
      }
    }
    n467 = case shown="Error" w1449 {
      selector: w1449 -> [w1474 _]
      tunnel: [w1474 errorcluster ? ("error out")] -> w1448
      frame #0 {
      }
      frame #1 {
        n468 = call "Display Message to User2"("Message"=string ?) -> ()  [unwired: 9 in, 2 out]
      }
    }
    n469 = case shown="Error" w1451 {
      selector: w1451 -> [w1477 _]
      tunnel: [w1477 errorcluster ? ("error out")] -> w1450
      frame #0 {
      }
      frame #1 {
        n470 = call "Display Message to User"("Message"=string ?) -> ()  [unwired: 9 in, 2 out]
      }
    }
    n471 = case shown="Error" w1447 {
      selector: w1447 -> [w1471 _]
      tunnel: [w1471 errorcluster ? ("error out")] -> w1446
      frame #0 {
      }
      frame #1 {
        n472 = call "Display Message to User3"("Message"=string ?) -> ()  [unwired: 9 in, 2 out]
      }
    }
    n473 = case shown="Error" w1442 {
      frame #0 {
      }
      frame #1 {
        n474 = call "Display Message to User15"("Message"=string ?) -> ()  [unwired: 9 in, 2 out]
      }
    }
    n475 = case shown="Error" w1445 {
      selector: w1445 -> [w1468 _]
      tunnel: [w1468 errorcluster ? ("error out")] -> w1441
      frame #0 {
      }
      frame #1 {
        n476 = call "Display Message to User4"("Message"=string ?) -> ()  [unwired: 9 in, 2 out]
      }
    }
    n477 = Get Notifier Status(notifier=w1439, error in (no error)=w1441) -> (notifier out=w1438:refnum<notifier>, current notification=w1437:bool, error out=w1440:errorcluster)  [unwired: 2 out]
  }
  n478 = Build Array(w66, w67, w68, w69) -> (w2:errorcluster[])
  n479 = call <vilib>:"Merge Errors.vi"("error array in"=w2) -> ("error out"=w86:errorcluster)  [unwired: 6 in]
  n480 = Build Array(w20, w19) -> (w6:errorcluster[])
  n481 = call <vilib>:"Merge Errors.vi"("error array in"=w6) -> ("error out"=w45:errorcluster)  [unwired: 6 in]
  n482 = Build Array(w26, w25) -> (w8:errorcluster[])
  n483 = call <vilib>:"Merge Errors.vi"("error array in"=w8) -> ("error out"=w43:errorcluster)  [unwired: 6 in]
  n484 = Build Array(w17, w16) -> (w5:errorcluster[])
  n485 = call <vilib>:"Merge Errors.vi"("error array in"=w5) -> ("error out"=w46:errorcluster)  [unwired: 6 in]
  n486 = Build Array(w52, w51) -> (w3:errorcluster[])
  n487 = call <vilib>:"Merge Errors.vi"("error array in"=w3) -> ("error out"=w50:errorcluster)  [unwired: 6 in]
  n488 = Build Array(w48, w47) -> (w4:errorcluster[])
  n489 = call <vilib>:"Merge Errors.vi"("error array in"=w4) -> ("error out"=w49:errorcluster)  [unwired: 6 in]
  n490 = Build Array(w23, w22) -> (w7:errorcluster[])
  n491 = call <vilib>:"Merge Errors.vi"("error array in"=w7) -> ("error out"=w44:errorcluster)  [unwired: 6 in]
  n492 = Build Array(w28, w27) -> (w9:errorcluster[])
  n493 = call <vilib>:"Merge Errors.vi"("error array in"=w9) -> ("error out"=w42:errorcluster)  [unwired: 6 in]
  n494 = Build Array(w30, w29) -> (w10:errorcluster[])
  n495 = call <vilib>:"Merge Errors.vi"("error array in"=w10) -> ("error out"=w41:errorcluster)  [unwired: 6 in]
  n496 = Build Array(w38, w37) -> (w12:errorcluster[])
  n497 = call <vilib>:"Merge Errors.vi"("error array in"=w12) -> ("error out"=w39:errorcluster)  [unwired: 6 in]
  n498 = Build Array(w36, w35) -> (w11:errorcluster[])
  n499 = call <vilib>:"Merge Errors.vi"("error array in"=w11) -> ("error out"=w40:errorcluster)  [unwired: 6 in]
  n500 = case shown="Error" w45 {
    selector: w45 -> [w1601 _]
    tunnel: [w1601 errorcluster ? ("error out")] -> w18
    frame #0 {
    }
    frame #1 {
      n501 = call "Display Message to User8"("Message"=string ?) -> ()  [unwired: 9 in, 2 out]
    }
  }
  n502 = case shown="Error" w43 {
    selector: w43 -> [w1604 _]
    tunnel: [w1604 errorcluster ? ("error out")] -> w24
    frame #0 {
    }
    frame #1 {
      n503 = call "Display Message to User10"("Message"=string ?) -> ()  [unwired: 9 in, 2 out]
    }
  }
  n504 = case shown="Error" w46 {
    selector: w46 -> [w1607 _]
    tunnel: [w1607 errorcluster ? ("error out")] -> w15
    frame #0 {
    }
    frame #1 {
      n505 = call "Display Message to User7"("Message"=string ?) -> ()  [unwired: 9 in, 2 out]
    }
  }
  n506 = case shown="Error" w50 {
    selector: w50 -> [w1610 _]
    tunnel: [w1610 errorcluster ? ("error out")] -> w13
    frame #0 {
    }
    frame #1 {
      n507 = call "Display Message to User5"("Message"=string ?) -> ()  [unwired: 9 in, 2 out]
    }
  }
  n508 = case shown="Error" w49 {
    selector: w49 -> [w1613 _]
    tunnel: [w1613 errorcluster ? ("error out")] -> w14
    frame #0 {
    }
    frame #1 {
      n509 = call "Display Message to User6"("Message"=string ?) -> ()  [unwired: 9 in, 2 out]
    }
  }
  n510 = case shown="Error" w44 {
    selector: w44 -> [w1616 _]
    tunnel: [w1616 errorcluster ? ("error out")] -> w21
    frame #0 {
    }
    frame #1 {
      n511 = call "Display Message to User9"("Message"=string ?) -> ()  [unwired: 9 in, 2 out]
    }
  }
  n512 = case shown="Error" w42 {
    selector: w42 -> [w1619 _]
    tunnel: [w1619 errorcluster ? ("error out")] -> w31
    frame #0 {
    }
    frame #1 {
      n513 = call "Display Message to User11"("Message"=string ?) -> ()  [unwired: 9 in, 2 out]
    }
  }
  n514 = case shown="Error" w41 {
    selector: w41 -> [w1622 _]
    tunnel: [w1622 errorcluster ? ("error out")] -> w32
    frame #0 {
    }
    frame #1 {
      n515 = call "Display Message to User12"("Message"=string ?) -> ()  [unwired: 9 in, 2 out]
    }
  }
  n516 = case shown="Error" w39 {
    selector: w39 -> [w1625 _]
    tunnel: [w1625 errorcluster ? ("error out")] -> w34
    frame #0 {
    }
    frame #1 {
      n517 = call "Display Message to User14"("Message"=string ?) -> ()  [unwired: 9 in, 2 out]
    }
  }
  n518 = case shown="Error" w40 {
    selector: w40 -> [w1628 _]
    tunnel: [w1628 errorcluster ? ("error out")] -> w33
    frame #0 {
    }
    frame #1 {
      n519 = call "Display Message to User13"("Message"=string ?) -> ()  [unwired: 9 in, 2 out]
    }
  }
  n520 = Build Array(w86, w34, w33, w32, w31, w24, w21, w18, w15, w14, w13) -> (w1:errorcluster[])
  n521 = call <vilib>:"Merge Errors.vi"("error array in"=w1) -> ("error out"=w56:errorcluster)  [unwired: 6 in]
  n522 = call <vilib>:"Simple Error Handler.vi"("error in (no error)"=w56) -> ("error out"=w57:errorcluster)  [unwired: 4 in, 4 out]
  n523 = call <vilib>:"Clear Errors.vi"("error in (no error)"=w57) -> ("error out"=w55:errorcluster)  [unwired: 6 in]
  n524 = Release Notifier(notifier=w62, force destroy? (F)=w58, error in (no error)=w55) -> (error out=w65:errorcluster)  [unwired: 2 out]
  n525 = Release Notifier(notifier=w61, force destroy? (F)=w58, error in (no error)=w65) -> (error out=w64:errorcluster)  [unwired: 2 out]
  n526 = Release Notifier(notifier=w60, force destroy? (F)=w58, error in (no error)=w64) -> (error out=w63:errorcluster)  [unwired: 2 out]
  n527 = Release Notifier(notifier=w59, force destroy? (F)=w58, error in (no error)=w63) -> (error out=w54:errorcluster)  [unwired: 2 out]
  n528 = call <vilib>:"Clear Errors.vi"("error in (no error)"=w54) -> ("error out"=w72:errorcluster)  [unwired: 6 in]
  n529 = property class="App"(error in=w72) -> (error out=w71:errorcluster, "App.Kind"=w70:T4)  [unwired: 1 in, 1 out]
  n530 = case shown="\"Run Time System\"" w70 {
    tunnel: w71 -> [_ _ _ _ _ _ _]
    frame #0 {
    }
    frame #1 {
    }
    frame #2 {
      n531 = Quit LabVIEW() -> ()  [unwired: 1 in]
    }
    frame #3 {
    }
    frame #4 {
    }
    frame #5 {
    }
    frame #6 {
    }
  }
